vi "Test JSON Parsing.vi"() -> ()   [LabVIEW 2018, in "InfluxDB Client.lvlib"]
uses:
  InfluxDB Client.lvlib
  <vilib>/LVH/i3 JSON/i3-json.lvlib
  Classes/Client/Client.lvclass
  Classes/Results/Results.lvclass
  Classes/Result/Result.lvclass
  Classes/Series/Series.lvclass
  Controls/TagSet.ctl
panel:
  out "Values":variant[][](array[variant])
  out "Error":string
  in  "Series index":i32
  in  "Results index":i32
  out "Statement_id":i32
  out "Series name":string
  out "Result partial":bool
  out "Series partial":bool
  out "Columns":string[](array[string])
  out "Tags":T1[](array[typedef])
  out "JSON":string="{\n  \"results\": [\n    {\n      \"statement_id\": 0,\n      \"series\": [\n        {\n          \"name\": \"ChunkTest\",\n          \"columns\": [\n            \"time\",\n            \"Val\"\n          ],\n          \"values\": [\n            [\n              1.5160504613572e+18,\n              0\n            ],\n            [\n              1.5160504613732e+18,\n              1\n            ],\n            [\n              1.5160504613892e+18,\n              2\n            ],\n            [\n              1.5160504614032e+18,\n              3\n            ],\n            [\n              1.5160504614187e+18,\n              4\n            ],\n            [\n              1.5160504614347e+18,\n              5\n            ],\n            [\n              1.5160504614511e+18,\n              6\n            ],\n            [\n              1.5160504614673e+18,\n              7\n            ],\n            [\n              1.5160504614824e+18,\n              8\n            ],\n            [\n              1.5160504614985e+18,\n              9\n            ]\n          ],\n          \"partial\": true\n        }\n      ],\n      \"partial\": true\n    }\n  ]\n}"
  # "rows"
  # "columns"
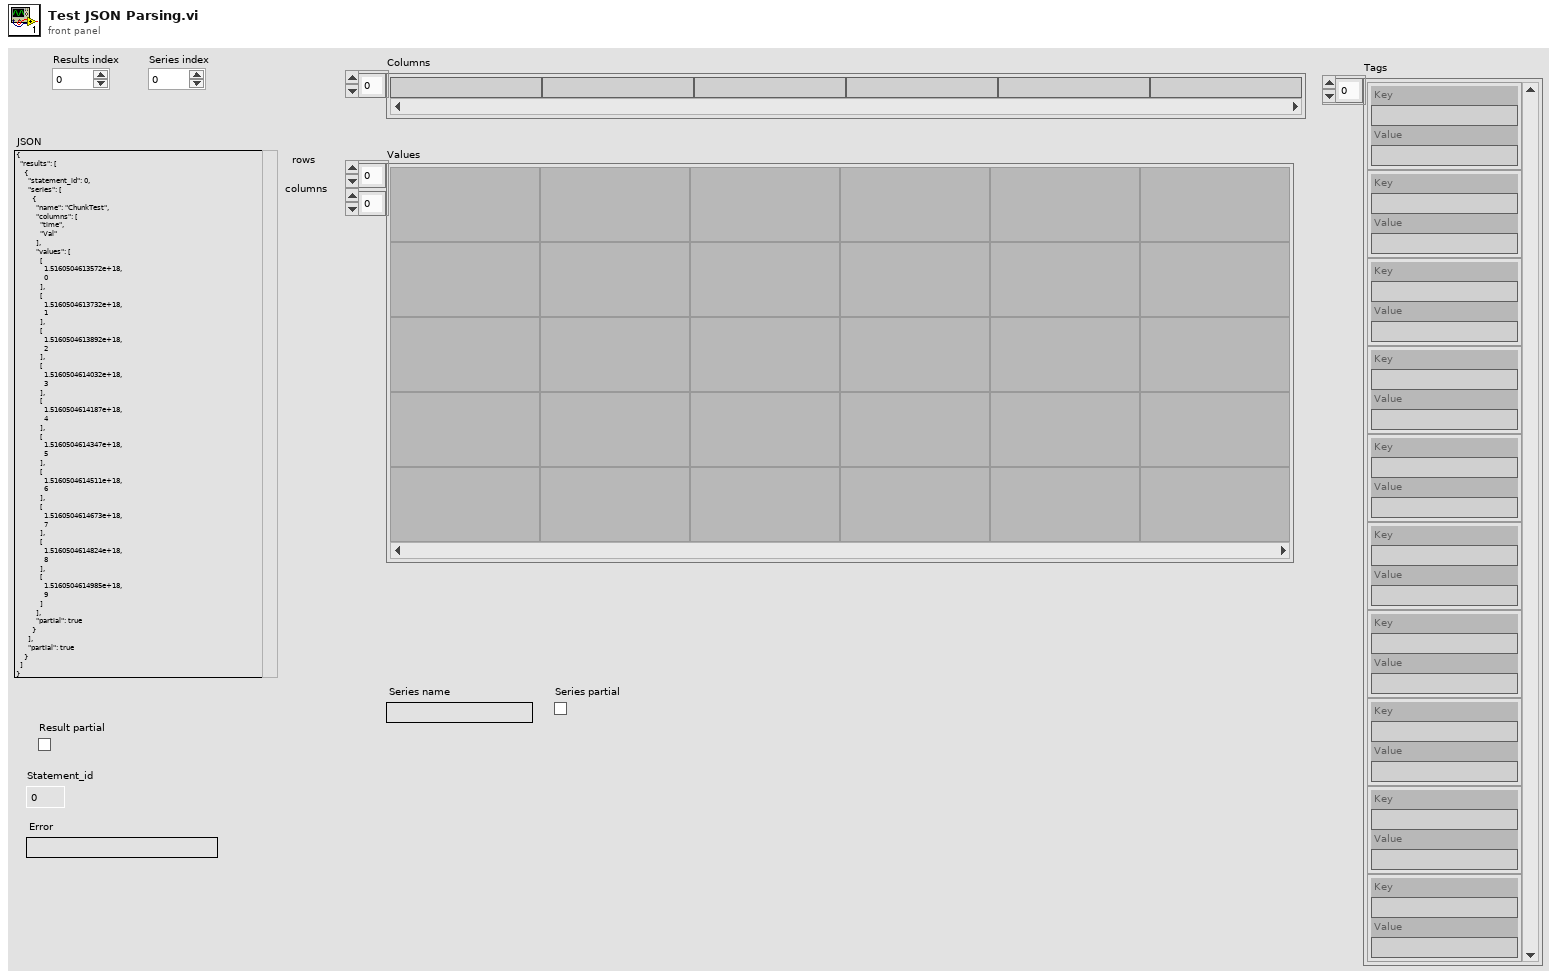
[diagram p1: front panel]
types:
  T1 = typedef "InfluxDB Client.lvlib/TagSet.ctl" = cluster{"Key":string, "Value":string}
  T2 = enum16{"open", "replace", "create", "open or create", "replace or create", "replace or create with confirmation"}
  T3 = typedef "Dictionary Object RefNum__ogtk.ctl" = refnum<k1>
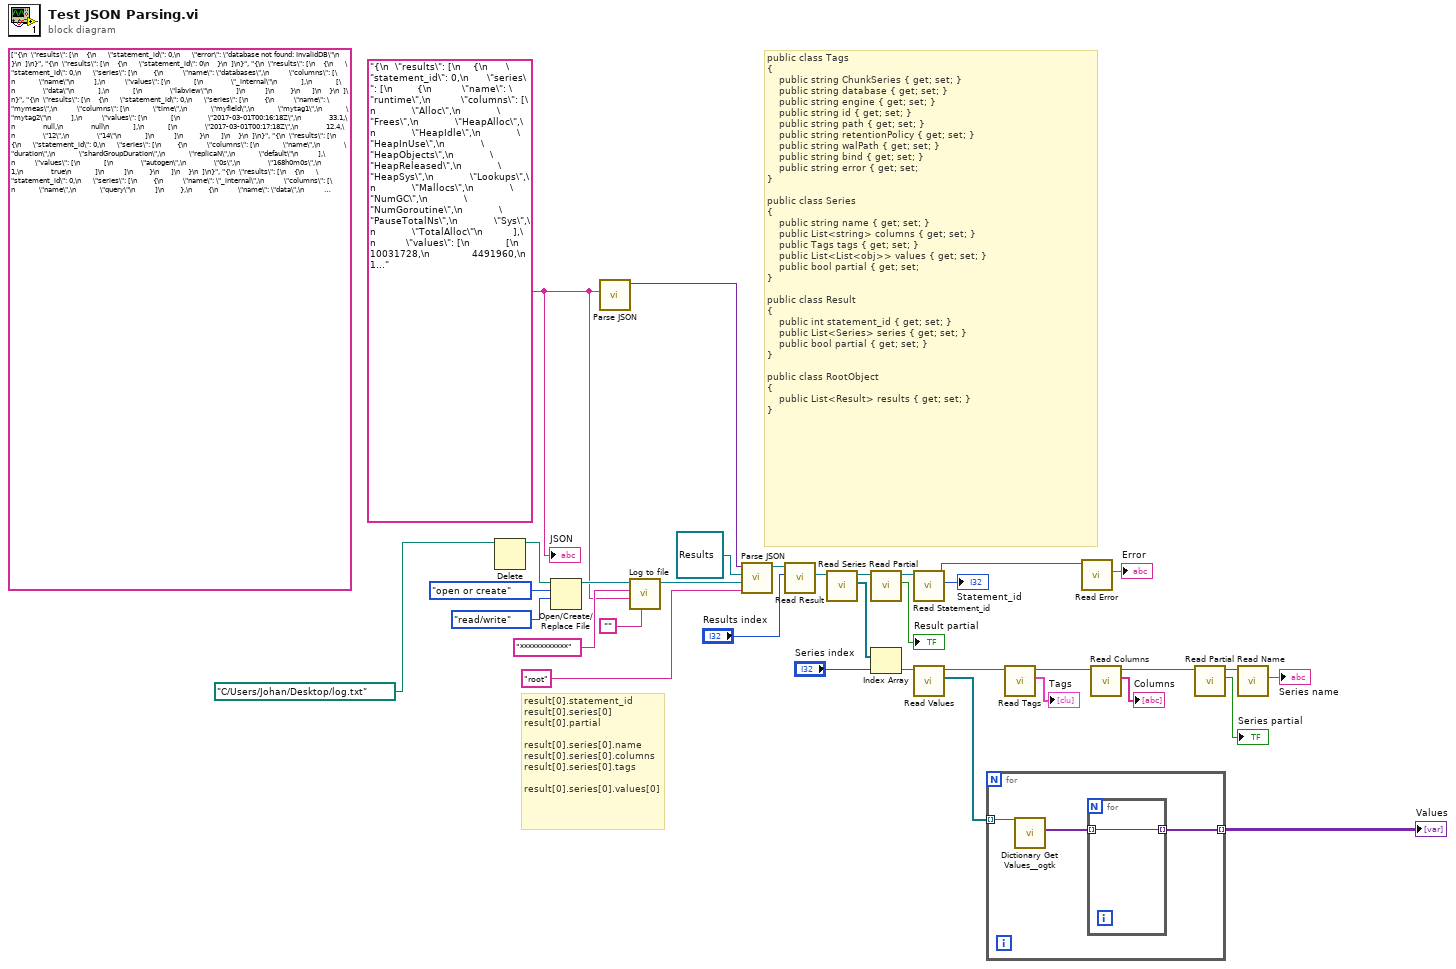
[diagram p0: block diagram]
diagram:
  w5 = "{\n  \"results\": [\n    {\n      \"statement_id\": 0,\n      \"series\": [\n        {\n          \"name\": \"runtime\",\n          \"columns\": [\n            \"Alloc\",\n            \"Frees\",\n            \"HeapAlloc\",\n            \"HeapIdle\",\n            \"HeapInUse\",\n            \"HeapObjects\",\n            \"HeapReleased\",\n            \"HeapSys\",\n            \"Lookups\",\n            \"Mallocs\",\n            \"NumGC\",\n            \"NumGoroutine\",\n            \"PauseTotalNs\",\n            \"Sys\",\n            \"TotalAlloc\"\n          ],\n          \"values\": [\n            [\n              10031728,\n              4491960,\n              10031728,\n              68689920,\n              12771328,\n              133250,\n              59473920,\n              81461248,\n              269,\n              4625210,\n              73,\n              27,\n              4009300,\n              89569528,\n              888359040\n            ]\n          ]\n        },\n        {\n          \"name\": \"queryExecutor\",\n          \"columns\": [\n            \"queriesActive\",\n            \"queriesExecuted\",\n            \"queriesFinished\",\n            \"queryDurationNs\",\n            \"recoveredPanics\"\n          ],\n          \"values\": [\n            [\n              1,\n              10,\n              9,\n              64001100,\n              0\n            ]\n          ]\n        },\n        {\n          \"name\": \"database\",\n          \"tags\": {\n            \"database\": \"_internal\"\n          },\n          \"columns\": [\n            \"numMeasurements\",\n            \"numSeries\"\n          ],\n          \"values\": [\n            [\n              12,\n              108\n            ]\n          ]\n        },\n        {\n          \"name\": \"database\",\n          \"tags\": {\n            \"database\": \"labview\"\n          },\n          \"columns\": [\n            \"numMeasurements\",\n            \"numSeries\"\n          ],\n          \"values\": [\n            [\n              1,\n              1\n            ]\n          ]\n        },\n        {\n          \"name\": \"database\",\n          \"tags\": {\n            \"database\": \"data\"\n          },\n          \"columns\": [\n            \"numMeasurements\",\n            \"numSeries\"\n          ],\n          \"values\": [\n            [\n              7,\n              23\n            ]\n          ]\n        },\n        {\n          \"name\": \"shard\",\n          \"tags\": {\n            \"database\": \"_internal\",\n            \"engine\": \"tsm1\",\n            \"id\": \"6\",\n            \"path\": \"C:\\\\Users\\\\Johan\\\\.influxdb\\\\data\\\\_internal\\\\monitor\\\\6\",\n            \"retentionPolicy\": \"monitor\",\n            \"walPath\": \"C:\\\\Users\\\\Johan\\\\.influxdb\\\\wal\\\\_internal\\\\monitor\\\\6\"\n          },\n          \"columns\": [\n            \"diskBytes\",\n            \"fieldsCreate\",\n            \"seriesCreate\",\n            \"writeBytes\",\n            \"writePointsDropped\",\n            \"writePointsErr\",\n            \"writePointsOk\",\n            \"writeReq\",\n            \"writeReqErr\",\n            \"writeReqOk\"\n          ],\n          \"values\": [\n            [\n              260046,\n              0,\n              109,\n              0,\n              0,\n              0,\n              0,\n              0,\n              0,\n              0\n            ]\n          ]\n        },\n        {\n          \"name\": \"tsm1_engine\",\n          \"tags\": {\n            \"database\": \"_internal\",\n            \"engine\": \"tsm1\",\n            \"id\": \"6\",\n            \"path\": \"C:\\\\Users\\\\Johan\\\\.influxdb\\\\data\\\\_internal\\\\monitor\\\\6\",\n            \"retentionPolicy\": \"monitor\",\n            \"walPath\": \"C:\\\\Users\\\\Johan\\\\.influxdb\\\\wal\\\\_internal\\\\monitor\\\\6\"\n          },\n          \"columns\": [\n            \"cacheCompactionDuration\",\n            \"cacheCompactionErr\",\n            \"cacheCompactions\",\n            \"cacheCompactionsActive\",\n            \"tsmFullCompactionDuration\",\n            \"tsmFullCompactionErr\",\n            \"tsmFullCompactionQueue\",\n            \"tsmFullCompactions\",\n            \"tsmFullCompactionsActive\",\n            \"tsmLevel1CompactionDuration\",\n            \"tsmLevel1CompactionErr\",\n            \"tsmLevel1CompactionQueue\",\n            \"tsmLevel1Compactions\",\n            \"tsmLevel1CompactionsActive\",\n            \"tsmLevel2CompactionDuration\",\n            \"tsmLevel2CompactionErr\",\n            \"tsmLevel2CompactionQueue\",\n            \"tsmLevel2Compactions\",\n            \"tsmLevel2CompactionsActive\",\n            \"tsmLevel3CompactionDuration\",\n            \"tsmLevel3CompactionErr\",\n            \"tsmLevel3CompactionQueue\",\n            \"tsmLevel3Compactions\",\n            \"tsmLevel3CompactionsActive\",\n            \"tsmOptimizeCompactionDuration\",\n            \"tsmOptimizeCompactionErr\",\n            \"tsmOptimizeCompactionQueue\",\n            \"tsmOptimizeCompactions\",\n            \"tsmOptimizeCompactionsActive\"\n          ],\n          \"values\": [\n            [\n              0,\n              0,\n              0,\n              0,\n              0,\n              0,\n              0,\n              0,\n              0,\n              0,\n              0,\n              0,\n              0,\n              0,\n              0,\n              0,\n              0,\n              0,\n              0,\n              0,\n              0,\n              0,\n              0,\n              0,\n              0,\n              0,\n              0,\n              0,\n              0\n            ]\n          ]\n        },\n        {\n          \"name\": \"tsm1_cache\",\n          \"tags\": {\n            \"database\": \"_internal\",\n            \"engine\": \"tsm1\",\n            \"id\": \"6\",\n            \"path\": \"C:\\\\Users\\\\Johan\\\\.influxdb\\\\data\\\\_internal\\\\monitor\\\\6\",\n            \"retentionPolicy\": \"monitor\",\n            \"walPath\": \"C:\\\\Users\\\\Johan\\\\.influxdb\\\\wal\\\\_internal\\\\monitor\\\\6\"\n          },\n          \"columns\": [\n            \"WALCompactionTimeMs\",\n            \"cacheAgeMs\",\n            \"cachedBytes\",\n            \"diskBytes\",\n            \"memBytes\",\n            \"snapshotCount\",\n            \"writeDropped\",\n            \"writeErr\",\n            \"writeOk\"\n          ],\n          \"values\": [\n            [\n              0,\n              0,\n              0,\n              0,\n              0,\n              0,\n              0,\n              0,\n              0\n            ]\n          ]\n        },\n        {\n          \"name\": \"tsm1_filestore\",\n          \"tags\": {\n            \"database\": \"_internal\",\n            \"engine\": \"tsm1\",\n            \"id\": \"6\",\n            \"path\": \"C:\\\\Users\\\\Johan\\\\.influxdb\\\\data\\\\_internal\\\\monitor\\\\6\",\n            \"retentionPolicy\": \"monitor\",\n            \"walPath\": \"C:\\\\Users\\\\Johan\\\\.influxdb\\\\wal\\\\_internal\\\\monitor\\\\6\"\n          },\n          \"columns\": [\n            \"diskBytes\",\n            \"numFiles\"\n          ],\n          \"values\": [\n            [\n              260046,\n              1\n            ]\n          ]\n        },\n        {\n          \"name\": \"tsm1_wal\",\n          \"tags\": {\n            \"database\": \"_internal\",\n            \"engine\": \"tsm1\",\n            \"id\": \"6\",\n            \"path\": \"C:\\\\Users\\\\Johan\\\\.influxdb\\\\data\\\\_internal\\\\monitor\\\\6\",\n            \"retentionPolicy\": \"monitor\",\n            \"walPath\": \"C:\\\\Users\\\\Johan\\\\.influxdb\\\\wal\\\\_internal\\\\monitor\\\\6\"\n          },\n          \"columns\": [\n            \"currentSegmentDiskBytes\",\n            \"oldSegmentsDiskBytes\",\n            \"writeErr\",\n            \"writeOk\"\n          ],\n          \"values\": [\n            [\n              0,\n              0,\n              0,\n              0\n            ]\n          ]\n        },\n        {\n          \"name\": \"shard\",\n          \"tags\": {\n            \"database\": \"data\",\n            \"engine\": \"tsm1\",\n            \"id\": \"10\",\n            \"path\": \"C:\\\\Users\\\\Johan\\\\.influxdb\\\\data\\\\data\\\\autogen\\\\10\",\n            \"retentionPolicy\": \"autogen\",\n            \"walPath\": \"C:\\\\Users\\\\Johan\\\\.influxdb\\\\wal\\\\data\\\\autogen\\\\10\"\n          },\n          \"columns\": [\n            \"diskBytes\",\n            \"fieldsCreate\",\n            \"seriesCreate\",\n            \"writeBytes\",\n            \"writePointsDropped\",\n            \"writePointsErr\",\n            \"writePointsOk\",\n            \"writeReq\",\n            \"writeReqErr\",\n            \"writeReqOk\"\n          ],\n          \"values\": [\n            [\n              614,\n              0,\n              23,\n              0,\n              0,\n              0,\n              0,\n              0,\n              0,\n              0\n            ]\n          ]\n        },\n        {\n          \"name\": \"tsm1_engine\",\n          \"tags\": {\n            \"database\": \"data\",\n            \"engine\": \"tsm1\",\n            \"id\": \"10\",\n            \"path\": \"C:\\\\Users\\\\Johan\\\\.influxdb\\\\data\\\\data\\\\autogen\\\\10\",\n            \"retentionPolicy\": \"autogen\",\n            \"walPath\": \"C:\\\\Users\\\\Johan\\\\.influxdb\\\\wal\\\\data\\\\autogen\\\\10\"\n          },\n          \"columns\": [\n            \"cacheCompactionDuration\",\n            \"cacheCompactionErr\",\n            \"cacheCompactions\",\n            \"cacheCompactionsActive\",\n            \"tsmFullCompactionDuration\",\n            \"tsmFullCompactionErr\",\n            \"tsmFullCompactionQueue\",\n            \"tsmFullCompactions\",\n            \"tsmFullCompactionsActive\",\n            \"tsmLevel1CompactionDuration\",\n            \"tsmLevel1CompactionErr\",\n            \"tsmLevel1CompactionQueue\",\n            \"tsmLevel1Compactions\",\n            \"tsmLevel1CompactionsActive\",\n            \"tsmLevel2CompactionDuration\",\n            \"tsmLevel2CompactionErr\",\n            \"tsmLevel2CompactionQueue\",\n            \"tsmLevel2Compactions\",\n            \"tsmLevel2CompactionsActive\",\n            \"tsmLevel3CompactionDuration\",\n            \"tsmLevel3CompactionErr\",\n            \"tsmLevel3CompactionQueue\",\n            \"tsmLevel3Compactions\",\n            \"tsmLevel3CompactionsActive\",\n            \"tsmOptimizeCompactionDuration\",\n            \"tsmOptimizeCompactionErr\",\n            \"tsmOptimizeCompactionQueue\",\n            \"tsmOptimizeCompactions\",\n            \"tsmOptimizeCompactionsActive\"\n          ],\n          \"values\": [\n            [\n              0,\n              0,\n              0,\n              0,\n              0,\n              0,\n              0,\n              0,\n              0,\n              0,\n              0,\n              0,\n              0,\n              0,\n              0,\n              0,\n              0,\n              0,\n              0,\n              0,\n              0,\n              0,\n              0,\n              0,\n              0,\n              0,\n              0,\n              0,\n              0\n            ]\n          ]\n        },\n        {\n          \"name\": \"tsm1_cache\",\n          \"tags\": {\n            \"database\": \"data\",\n            \"engine\": \"tsm1\",\n            \"id\": \"10\",\n            \"path\": \"C:\\\\Users\\\\Johan\\\\.influxdb\\\\data\\\\data\\\\autogen\\\\10\",\n            \"retentionPolicy\": \"autogen\",\n            \"walPath\": \"C:\\\\Users\\\\Johan\\\\.influxdb\\\\wal\\\\data\\\\autogen\\\\10\"\n          },\n          \"columns\": [\n            \"WALCompactionTimeMs\",\n            \"cacheAgeMs\",\n            \"cachedBytes\",\n            \"diskBytes\",\n            \"memBytes\",\n            \"snapshotCount\",\n            \"writeDropped\",\n            \"writeErr\",\n            \"writeOk\"\n          ],\n          \"values\": [\n            [\n              0,\n              0,\n              0,\n              0,\n              0,\n              0,\n              0,\n              0,\n              0\n            ]\n          ]\n        },\n        {\n          \"name\": \"tsm1_filestore\",\n          \"tags\": {\n            \"database\": \"data\",\n            \"engine\": \"tsm1\",\n            \"id\": \"10\",\n            \"path\": \"C:\\\\Users\\\\Johan\\\\.influxdb\\\\data\\\\data\\\\autogen\\\\10\",\n            \"retentionPolicy\": \"autogen\",\n            \"walPath\": \"C:\\\\Users\\\\Johan\\\\.influxdb\\\\wal\\\\data\\\\autogen\\\\10\"\n          },\n          \"columns\": [\n            \"diskBytes\",\n            \"numFiles\"\n          ],\n          \"values\": [\n            [\n              614,\n              1\n            ]\n          ]\n        },\n        {\n          \"name\": \"tsm1_wal\",\n          \"tags\": {\n            \"database\": \"data\",\n            \"engine\": \"tsm1\",\n            \"id\": \"10\",\n            \"path\": \"C:\\\\Users\\\\Johan\\\\.influxdb\\\\data\\\\data\\\\autogen\\\\10\",\n            \"retentionPolicy\": \"autogen\",\n            \"walPath\": \"C:\\\\Users\\\\Johan\\\\.influxdb\\\\wal\\\\data\\\\autogen\\\\10\"\n          },\n          \"columns\": [\n            \"currentSegmentDiskBytes\",\n            \"oldSegmentsDiskBytes\",\n            \"writeErr\",\n            \"writeOk\"\n          ],\n          \"values\": [\n            [\n              0,\n              0,\n              0,\n              0\n            ]\n          ]\n        },\n        {\n          \"name\": \"shard\",\n          \"tags\": {\n            \"database\": \"data\",\n            \"engine\": \"tsm1\",\n            \"id\": \"11\",\n            \"path\": \"C:\\\\Users\\\\Johan\\\\.influxdb\\\\data\\\\data\\\\autogen\\\\11\",\n            \"retentionPolicy\": \"autogen\",\n            \"walPath\": \"C:\\\\Users\\\\Johan\\\\.influxdb\\\\wal\\\\data\\\\autogen\\\\11\"\n          },\n          \"columns\": [\n            \"diskBytes\",\n            \"fieldsCreate\",\n            \"seriesCreate\",\n            \"writeBytes\",\n            \"writePointsDropped\",\n            \"writePointsErr\",\n            \"writePointsOk\",\n            \"writeReq\",\n            \"writeReqErr\",\n            \"writeReqOk\"\n          ],\n          \"values\": [\n            [\n              115,\n              0,\n              23,\n              0,\n              0,\n              0,\n              0,\n              0,\n              0,\n              0\n            ]\n          ]\n        },\n        {\n          \"name\": \"tsm1_engine\",\n          \"tags\": {\n            \"database\": \"data\",\n            \"engine\": \"tsm1\",\n            \"id\": \"11\",\n            \"path\": \"C:\\\\Users\\\\Johan\\\\.influxdb\\\\data\\\\data\\\\autogen\\\\11\",\n            \"retentionPolicy\": \"autogen\",\n            \"walPath\": \"C:\\\\Users\\\\Johan\\\\.influxdb\\\\wal\\\\data\\\\autogen\\\\11\"\n          },\n          \"columns\": [\n            \"cacheCompactionDuration\",\n            \"cacheCompactionErr\",\n            \"cacheCompactions\",\n            \"cacheCompactionsActive\",\n            \"tsmFullCompactionDuration\",\n            \"tsmFullCompactionErr\",\n            \"tsmFullCompactionQueue\",\n            \"tsmFullCompactions\",\n            \"tsmFullCompactionsActive\",\n            \"tsmLevel1CompactionDuration\",\n            \"tsmLevel1CompactionErr\",\n            \"tsmLevel1CompactionQueue\",\n            \"tsmLevel1Compactions\",\n            \"tsmLevel1CompactionsActive\",\n            \"tsmLevel2CompactionDuration\",\n            \"tsmLevel2CompactionErr\",\n            \"tsmLevel2CompactionQueue\",\n            \"tsmLevel2Compactions\",\n            \"tsmLevel2CompactionsActive\",\n            \"tsmLevel3CompactionDuration\",\n            \"tsmLevel3CompactionErr\",\n            \"tsmLevel3CompactionQueue\",\n            \"tsmLevel3Compactions\",\n            \"tsmLevel3CompactionsActive\",\n            \"tsmOptimizeCompactionDuration\",\n            \"tsmOptimizeCompactionErr\",\n            \"tsmOptimizeCompactionQueue\",\n            \"tsmOptimizeCompactions\",\n            \"tsmOptimizeCompactionsActive\"\n          ],\n          \"values\": [\n            [\n              0,\n              0,\n              0,\n              0,\n              0,\n              0,\n              0,\n              0,\n              0,\n              0,\n              0,\n              0,\n              0,\n              0,\n              0,\n              0,\n              0,\n              0,\n              0,\n              0,\n              0,\n              0,\n              0,\n              0,\n              0,\n              0,\n              0,\n              0,\n              0\n            ]\n          ]\n        },\n        {\n          \"name\": \"tsm1_cache\",\n          \"tags\": {\n            \"database\": \"data\",\n            \"engine\": \"tsm1\",\n            \"id\": \"11\",\n            \"path\": \"C:\\\\Users\\\\Johan\\\\.influxdb\\\\data\\\\data\\\\autogen\\\\11\",\n            \"retentionPolicy\": \"autogen\",\n            \"walPath\": \"C:\\\\Users\\\\Johan\\\\.influxdb\\\\wal\\\\data\\\\autogen\\\\11\"\n          },\n          \"columns\": [\n            \"WALCompactionTimeMs\",\n            \"cacheAgeMs\",\n            \"cachedBytes\",\n            \"diskBytes\",\n            \"memBytes\",\n            \"snapshotCount\",\n            \"writeDropped\",\n            \"writeErr\",\n            \"writeOk\"\n          ],\n          \"values\": [\n            [\n              0,\n              0,\n              0,\n              0,\n              0,\n              0,\n              0,\n              0,\n              0\n            ]\n          ]\n        },\n        {\n          \"name\": \"tsm1_filestore\",\n          \"tags\": {\n            \"database\": \"data\",\n            \"engine\": \"tsm1\",\n            \"id\": \"11\",\n            \"path\": \"C:\\\\Users\\\\Johan\\\\.influxdb\\\\data\\\\data\\\\autogen\\\\11\",\n            \"retentionPolicy\": \"autogen\",\n            \"walPath\": \"C:\\\\Users\\\\Johan\\\\.influxdb\\\\wal\\\\data\\\\autogen\\\\11\"\n          },\n          \"columns\": [\n            \"diskBytes\",\n            \"numFiles\"\n          ],\n          \"values\": [\n            [\n              115,\n              1\n            ]\n          ]\n        },\n        {\n          \"name\": \"tsm1_wal\",\n          \"tags\": {\n            \"database\": \"data\",\n            \"engine\": \"tsm1\",\n            \"id\": \"11\",\n            \"path\": \"C:\\\\Users\\\\Johan\\\\.influxdb\\\\data\\\\data\\\\autogen\\\\11\",\n            \"retentionPolicy\": \"autogen\",\n            \"walPath\": \"C:\\\\Users\\\\Johan\\\\.influxdb\\\\wal\\\\data\\\\autogen\\\\11\"\n          },\n          \"columns\": [\n            \"currentSegmentDiskBytes\",\n            \"oldSegmentsDiskBytes\",\n            \"writeErr\",\n            \"writeOk\"\n          ],\n          \"values\": [\n            [\n              0,\n              0,\n              0,\n              0\n            ]\n          ]\n        },\n        {\n          \"name\": \"shard\",\n          \"tags\": {\n            \"database\": \"data\",\n            \"engine\": \"tsm1\",\n            \"id\": \"12\",\n            \"path\": \"C:\\\\Users\\\\Johan\\\\.influxdb\\\\data\\\\data\\\\autogen\\\\12\",\n            \"retentionPolicy\": \"autogen\",\n            \"walPath\": \"C:\\\\Users\\\\Johan\\\\.influxdb\\\\wal\\\\data\\\\autogen\\\\12\"\n          },\n          \"columns\": [\n            \"diskBytes\",\n            \"fieldsCreate\",\n            \"seriesCreate\",\n            \"writeBytes\",\n            \"writePointsDropped\",\n            \"writePointsErr\",\n            \"writePointsOk\",\n            \"writeReq\",\n            \"writeReqErr\",\n            \"writeReqOk\"\n          ],\n          \"values\": [\n            [\n              58924,\n              0,\n              23,\n              0,\n              0,\n              0,\n              0,\n              0,\n              0,\n              0\n            ]\n          ]\n        },\n        {\n          \"name\": \"tsm1_engine\",\n          \"tags\": {\n            \"database\": \"data\",\n            \"engine\": \"tsm1\",\n            \"id\": \"12\",\n            \"path\": \"C:\\\\Users\\\\Johan\\\\.influxdb\\\\data\\\\data\\\\autogen\\\\12\",\n            \"retentionPolicy\": \"autogen\",\n            \"walPath\": \"C:\\\\Users\\\\Johan\\\\.influxdb\\\\wal\\\\data\\\\autogen\\\\12\"\n          },\n          \"columns\": [\n            \"cacheCompactionDuration\",\n            \"cacheCompactionErr\",\n            \"cacheCompactions\",\n            \"cacheCompactionsActive\",\n            \"tsmFullCompactionDuration\",\n            \"tsmFullCompactionErr\",\n            \"tsmFullCompactionQueue\",\n            \"tsmFullCompactions\",\n            \"tsmFullCompactionsActive\",\n            \"tsmLevel1CompactionDuration\",\n            \"tsmLevel1CompactionErr\",\n            \"tsmLevel1CompactionQueue\",\n            \"tsmLevel1Compactions\",\n            \"tsmLevel1CompactionsActive\",\n            \"tsmLevel2CompactionDuration\",\n            \"tsmLevel2CompactionErr\",\n            \"tsmLevel2CompactionQueue\",\n            \"tsmLevel2Compactions\",\n            \"tsmLevel2CompactionsActive\",\n            \"tsmLevel3CompactionDuration\",\n            \"tsmLevel3CompactionErr\",\n            \"tsmLevel3CompactionQueue\",\n            \"tsmLevel3Compactions\",\n            \"tsmLevel3CompactionsActive\",\n            \"tsmOptimizeCompactionDuration\",\n            \"tsmOptimizeCompactionErr\",\n            \"tsmOptimizeCompactionQueue\",\n            \"tsmOptimizeCompactions\",\n            \"tsmOptimizeCompactionsActive\"\n          ],\n          \"values\": [\n            [\n              0,\n              0,\n              0,\n              0,\n              0,\n              0,\n              0,\n              0,\n              0,\n              0,\n              0,\n              0,\n              0,\n              0,\n              0,\n              0,\n              0,\n              0,\n              0,\n              0,\n              0,\n              0,\n              0,\n              0,\n              0,\n              0,\n              0,\n              0,\n              0\n            ]\n          ]\n        },\n        {\n          \"name\": \"tsm1_cache\",\n          \"tags\": {\n            \"database\": \"data\",\n            \"engine\": \"tsm1\",\n            \"id\": \"12\",\n            \"path\": \"C:\\\\Users\\\\Johan\\\\.influxdb\\\\data\\\\data\\\\autogen\\\\12\",\n            \"retentionPolicy\": \"autogen\",\n            \"walPath\": \"C:\\\\Users\\\\Johan\\\\.influxdb\\\\wal\\\\data\\\\autogen\\\\12\"\n          },\n          \"columns\": [\n            \"WALCompactionTimeMs\",\n            \"cacheAgeMs\",\n            \"cachedBytes\",\n            \"diskBytes\",\n            \"memBytes\",\n            \"snapshotCount\",\n            \"writeDropped\",\n            \"writeErr\",\n            \"writeOk\"\n          ],\n          \"values\": [\n            [\n              0,\n              0,\n              0,\n              0,\n              0,\n              0,\n              0,\n              0,\n              0\n            ]\n          ]\n        },\n        {\n          \"name\": \"tsm1_filestore\",\n          \"tags\": {\n            \"database\": \"data\",\n            \"engine\": \"tsm1\",\n            \"id\": \"12\",\n            \"path\": \"C:\\\\Users\\\\Johan\\\\.influxdb\\\\data\\\\data\\\\autogen\\\\12\",\n            \"retentionPolicy\": \"autogen\",\n            \"walPath\": \"C:\\\\Users\\\\Johan\\\\.influxdb\\\\wal\\\\data\\\\autogen\\\\12\"\n          },\n          \"columns\": [\n            \"diskBytes\",\n            \"numFiles\"\n          ],\n          \"values\": [\n            [\n              58924,\n              1\n            ]\n          ]\n        },\n        {\n          \"name\": \"tsm1_wal\",\n          \"tags\": {\n            \"database\": \"data\",\n            \"engine\": \"tsm1\",\n            \"id\": \"12\",\n            \"path\": \"C:\\\\Users\\\\Johan\\\\.influxdb\\\\data\\\\data\\\\autogen\\\\12\",\n            \"retentionPolicy\": \"autogen\",\n            \"walPath\": \"C:\\\\Users\\\\Johan\\\\.influxdb\\\\wal\\\\data\\\\autogen\\\\12\"\n          },\n          \"columns\": [\n            \"currentSegmentDiskBytes\",\n            \"oldSegmentsDiskBytes\",\n            \"writeErr\",\n            \"writeOk\"\n          ],\n          \"values\": [\n            [\n              0,\n              0,\n              0,\n              0\n            ]\n          ]\n        },\n        {\n          \"name\": \"shard\",\n          \"tags\": {\n            \"database\": \"_internal\",\n            \"engine\": \"tsm1\",\n            \"id\": \"13\",\n            \"path\": \"C:\\\\Users\\\\Johan\\\\.influxdb\\\\data\\\\_internal\\\\monitor\\\\13\",\n            \"retentionPolicy\": \"monitor\",\n            \"walPath\": \"C:\\\\Users\\\\Johan\\\\.influxdb\\\\wal\\\\_internal\\\\monitor\\\\13\"\n          },\n          \"columns\": [\n            \"diskBytes\",\n            \"fieldsCreate\",\n            \"seriesCreate\",\n            \"writeBytes\",\n            \"writePointsDropped\",\n            \"writePointsErr\",\n            \"writePointsOk\",\n            \"writeReq\",\n            \"writeReqErr\",\n            \"writeReqOk\"\n          ],\n          \"values\": [\n            [\n              157086,\n              0,\n              109,\n              0,\n              0,\n              0,\n              0,\n              0,\n              0,\n              0\n            ]\n          ]\n        },\n        {\n          \"name\": \"tsm1_engine\",\n          \"tags\": {\n            \"database\": \"_internal\",\n            \"engine\": \"tsm1\",\n            \"id\": \"13\",\n            \"path\": \"C:\\\\Users\\\\Johan\\\\.influxdb\\\\data\\\\_internal\\\\monitor\\\\13\",\n            \"retentionPolicy\": \"monitor\",\n            \"walPath\": \"C:\\\\Users\\\\Johan\\\\.influxdb\\\\wal\\\\_internal\\\\monitor\\\\13\"\n          },\n          \"columns\": [\n            \"cacheCompactionDuration\",\n            \"cacheCompactionErr\",\n            \"cacheCompactions\",\n            \"cacheCompactionsActive\",\n            \"tsmFullCompactionDuration\",\n            \"tsmFullCompactionErr\",\n            \"tsmFullCompactionQueue\",\n            \"tsmFullCompactions\",\n            \"tsmFullCompactionsActive\",\n            \"tsmLevel1CompactionDuration\",\n            \"tsmLevel1CompactionErr\",\n            \"tsmLevel1CompactionQueue\",\n            \"tsmLevel1Compactions\",\n            \"tsmLevel1CompactionsActive\",\n            \"tsmLevel2CompactionDuration\",\n            \"tsmLevel2CompactionErr\",\n            \"tsmLevel2CompactionQueue\",\n            \"tsmLevel2Compactions\",\n            \"tsmLevel2CompactionsActive\",\n            \"tsmLevel3CompactionDuration\",\n            \"tsmLevel3CompactionErr\",\n            \"tsmLevel3CompactionQueue\",\n            \"tsmLevel3Compactions\",\n            \"tsmLevel3CompactionsActive\",\n            \"tsmOptimizeCompactionDuration\",\n            \"tsmOptimizeCompactionErr\",\n            \"tsmOptimizeCompactionQueue\",\n            \"tsmOptimizeCompactions\",\n            \"tsmOptimizeCompactionsActive\"\n          ],\n          \"values\": [\n            [\n              0,\n              0,\n              0,\n              0,\n              0,\n              0,\n              0,\n              0,\n              0,\n              0,\n              0,\n              0,\n              0,\n              0,\n              0,\n              0,\n              0,\n              0,\n              0,\n              0,\n              0,\n              0,\n              0,\n              0,\n              0,\n              0,\n              0,\n              0,\n              0\n            ]\n          ]\n        },\n        {\n          \"name\": \"tsm1_cache\",\n          \"tags\": {\n            \"database\": \"_internal\",\n            \"engine\": \"tsm1\",\n            \"id\": \"13\",\n            \"path\": \"C:\\\\Users\\\\Johan\\\\.influxdb\\\\data\\\\_internal\\\\monitor\\\\13\",\n            \"retentionPolicy\": \"monitor\",\n            \"walPath\": \"C:\\\\Users\\\\Johan\\\\.influxdb\\\\wal\\\\_internal\\\\monitor\\\\13\"\n          },\n          \"columns\": [\n            \"WALCompactionTimeMs\",\n            \"cacheAgeMs\",\n            \"cachedBytes\",\n            \"diskBytes\",\n            \"memBytes\",\n            \"snapshotCount\",\n            \"writeDropped\",\n            \"writeErr\",\n            \"writeOk\"\n          ],\n          \"values\": [\n            [\n              0,\n              0,\n              0,\n              0,\n              0,\n              0,\n              0,\n              0,\n              0\n            ]\n          ]\n        },\n        {\n          \"name\": \"tsm1_filestore\",\n          \"tags\": {\n            \"database\": \"_internal\",\n            \"engine\": \"tsm1\",\n            \"id\": \"13\",\n            \"path\": \"C:\\\\Users\\\\Johan\\\\.influxdb\\\\data\\\\_internal\\\\monitor\\\\13\",\n            \"retentionPolicy\": \"monitor\",\n            \"walPath\": \"C:\\\\Users\\\\Johan\\\\.influxdb\\\\wal\\\\_internal\\\\monitor\\\\13\"\n          },\n          \"columns\": [\n            \"diskBytes\",\n            \"numFiles\"\n          ],\n          \"values\": [\n            [\n              157086,\n              1\n            ]\n          ]\n        },\n        {\n          \"name\": \"tsm1_wal\",\n          \"tags\": {\n            \"database\": \"_internal\",\n            \"engine\": \"tsm1\",\n            \"id\": \"13\",\n            \"path\": \"C:\\\\Users\\\\Johan\\\\.influxdb\\\\data\\\\_internal\\\\monitor\\\\13\",\n            \"retentionPolicy\": \"monitor\",\n            \"walPath\": \"C:\\\\Users\\\\Johan\\\\.influxdb\\\\wal\\\\_internal\\\\monitor\\\\13\"\n          },\n          \"columns\": [\n            \"currentSegmentDiskBytes\",\n            \"oldSegmentsDiskBytes\",\n            \"writeErr\",\n            \"writeOk\"\n          ],\n          \"values\": [\n            [\n              0,\n              0,\n              0,\n              0\n            ]\n          ]\n        },\n        {\n          \"name\": \"shard\",\n          \"tags\": {\n            \"database\": \"_internal\",\n            \"engine\": \"tsm1\",\n            \"id\": \"14\",\n            \"path\": \"C:\\\\Users\\\\Johan\\\\.influxdb\\\\data\\\\_internal\\\\monitor\\\\14\",\n            \"retentionPolicy\": \"monitor\",\n            \"walPath\": \"C:\\\\Users\\\\Johan\\\\.influxdb\\\\wal\\\\_internal\\\\monitor\\\\14\"\n          },\n          \"columns\": [\n            \"diskBytes\",\n            \"fieldsCreate\",\n            \"seriesCreate\",\n            \"writeBytes\",\n            \"writePointsDropped\",\n            \"writePointsErr\",\n            \"writePointsOk\",\n            \"writeReq\",\n            \"writeReqErr\",\n            \"writeReqOk\"\n          ],\n          \"values\": [\n            [\n              306311,\n              0,\n              109,\n              0,\n              0,\n              0,\n              0,\n              0,\n              0,\n              0\n            ]\n          ]\n        },\n        {\n          \"name\": \"tsm1_engine\",\n          \"tags\": {\n            \"database\": \"_internal\",\n            \"engine\": \"tsm1\",\n            \"id\": \"14\",\n            \"path\": \"C:\\\\Users\\\\Johan\\\\.influxdb\\\\data\\\\_internal\\\\monitor\\\\14\",\n            \"retentionPolicy\": \"monitor\",\n            \"walPath\": \"C:\\\\Users\\\\Johan\\\\.influxdb\\\\wal\\\\_internal\\\\monitor\\\\14\"\n          },\n          \"columns\": [\n            \"cacheCompactionDuration\",\n            \"cacheCompactionErr\",\n            \"cacheCompactions\",\n            \"cacheCompactionsActive\",\n            \"tsmFullCompactionDuration\",\n            \"tsmFullCompactionErr\",\n            \"tsmFullCompactionQueue\",\n            \"tsmFullCompactions\",\n            \"tsmFullCompactionsActive\",\n            \"tsmLevel1CompactionDuration\",\n            \"tsmLevel1CompactionErr\",\n            \"tsmLevel1CompactionQueue\",\n            \"tsmLevel1Compactions\",\n            \"tsmLevel1CompactionsActive\",\n            \"tsmLevel2CompactionDuration\",\n            \"tsmLevel2CompactionErr\",\n            \"tsmLevel2CompactionQueue\",\n            \"tsmLevel2Compactions\",\n            \"tsmLevel2CompactionsActive\",\n            \"tsmLevel3CompactionDuration\",\n            \"tsmLevel3CompactionErr\",\n            \"tsmLevel3CompactionQueue\",\n            \"tsmLevel3Compactions\",\n            \"tsmLevel3CompactionsActive\",\n            \"tsmOptimizeCompactionDuration\",\n            \"tsmOptimizeCompactionErr\",\n            \"tsmOptimizeCompactionQueue\",\n            \"tsmOptimizeCompactions\",\n            \"tsmOptimizeCompactionsActive\"\n          ],\n          \"values\": [\n            [\n              0,\n              0,\n              0,\n              0,\n              0,\n              0,\n              0,\n              0,\n              0,\n              0,\n              0,\n              0,\n              0,\n              0,\n              0,\n              0,\n              0,\n              0,\n              0,\n              0,\n              0,\n              0,\n              0,\n              0,\n              0,\n              0,\n              0,\n              0,\n              0\n            ]\n          ]\n        },\n        {\n          \"name\": \"tsm1_cache\",\n          \"tags\": {\n            \"database\": \"_internal\",\n            \"engine\": \"tsm1\",\n            \"id\": \"14\",\n            \"path\": \"C:\\\\Users\\\\Johan\\\\.influxdb\\\\data\\\\_internal\\\\monitor\\\\14\",\n            \"retentionPolicy\": \"monitor\",\n            \"walPath\": \"C:\\\\Users\\\\Johan\\\\.influxdb\\\\wal\\\\_internal\\\\monitor\\\\14\"\n          },\n          \"columns\": [\n            \"WALCompactionTimeMs\",\n            \"cacheAgeMs\",\n            \"cachedBytes\",\n            \"diskBytes\",\n            \"memBytes\",\n            \"snapshotCount\",\n            \"writeDropped\",\n            \"writeErr\",\n            \"writeOk\"\n          ],\n          \"values\": [\n            [\n              0,\n              0,\n              0,\n              0,\n              0,\n              0,\n              0,\n              0,\n              0\n            ]\n          ]\n        },\n        {\n          \"name\": \"tsm1_filestore\",\n          \"tags\": {\n            \"database\": \"_internal\",\n            \"engine\": \"tsm1\",\n            \"id\": \"14\",\n            \"path\": \"C:\\\\Users\\\\Johan\\\\.influxdb\\\\data\\\\_internal\\\\monitor\\\\14\",\n            \"retentionPolicy\": \"monitor\",\n            \"walPath\": \"C:\\\\Users\\\\Johan\\\\.influxdb\\\\wal\\\\_internal\\\\monitor\\\\14\"\n          },\n          \"columns\": [\n            \"diskBytes\",\n            \"numFiles\"\n          ],\n          \"values\": [\n            [\n              306311,\n              1\n            ]\n          ]\n        },\n        {\n          \"name\": \"tsm1_wal\",\n          \"tags\": {\n            \"database\": \"_internal\",\n            \"engine\": \"tsm1\",\n            \"id\": \"14\",\n            \"path\": \"C:\\\\Users\\\\Johan\\\\.influxdb\\\\data\\\\_internal\\\\monitor\\\\14\",\n            \"retentionPolicy\": \"monitor\",\n            \"walPath\": \"C:\\\\Users\\\\Johan\\\\.influxdb\\\\wal\\\\_internal\\\\monitor\\\\14\"\n          },\n          \"columns\": [\n            \"currentSegmentDiskBytes\",\n            \"oldSegmentsDiskBytes\",\n            \"writeErr\",\n            \"writeOk\"\n          ],\n          \"values\": [\n            [\n              0,\n              0,\n              0,\n              0\n            ]\n          ]\n        },\n        {\n          \"name\": \"shard\",\n          \"tags\": {\n            \"database\": \"_internal\",\n            \"engine\": \"tsm1\",\n            \"id\": \"15\",\n            \"path\": \"C:\\\\Users\\\\Johan\\\\.influxdb\\\\data\\\\_internal\\\\monitor\\\\15\",\n            \"retentionPolicy\": \"monitor\",\n            \"walPath\": \"C:\\\\Users\\\\Johan\\\\.influxdb\\\\wal\\\\_internal\\\\monitor\\\\15\"\n          },\n          \"columns\": [\n            \"diskBytes\",\n            \"fieldsCreate\",\n            \"seriesCreate\",\n            \"writeBytes\",\n            \"writePointsDropped\",\n            \"writePointsErr\",\n            \"writePointsOk\",\n            \"writeReq\",\n            \"writeReqErr\",\n            \"writeReqOk\"\n          ],\n          \"values\": [\n            [\n              697298,\n              0,\n              109,\n              0,\n              0,\n              0,\n              0,\n              0,\n              0,\n              0\n            ]\n          ]\n        },\n        {\n          \"name\": \"tsm1_engine\",\n          \"tags\": {\n            \"database\": \"_internal\",\n            \"engine\": \"tsm1\",\n            \"id\": \"15\",\n            \"path\": \"C:\\\\Users\\\\Johan\\\\.influxdb\\\\data\\\\_internal\\\\monitor\\\\15\",\n            \"retentionPolicy\": \"monitor\",\n            \"walPath\": \"C:\\\\Users\\\\Johan\\\\.influxdb\\\\wal\\\\_internal\\\\monitor\\\\15\"\n          },\n          \"columns\": [\n            \"cacheCompactionDuration\",\n            \"cacheCompactionErr\",\n            \"cacheCompactions\",\n            \"cacheCompactionsActive\",\n            \"tsmFullCompactionDuration\",\n            \"tsmFullCompactionErr\",\n            \"tsmFullCompactionQueue\",\n            \"tsmFullCompactions\",\n            \"tsmFullCompactionsActive\",\n            \"tsmLevel1CompactionDuration\",\n            \"tsmLevel1CompactionErr\",\n            \"tsmLevel1CompactionQueue\",\n            \"tsmLevel1Compactions\",\n            \"tsmLevel1CompactionsActive\",\n            \"tsmLevel2CompactionDuration\",\n            \"tsmLevel2CompactionErr\",\n            \"tsmLevel2CompactionQueue\",\n            \"tsmLevel2Compactions\",\n            \"tsmLevel2CompactionsActive\",\n            \"tsmLevel3CompactionDuration\",\n            \"tsmLevel3CompactionErr\",\n            \"tsmLevel3CompactionQueue\",\n            \"tsmLevel3Compactions\",\n            \"tsmLevel3CompactionsActive\",\n            \"tsmOptimizeCompactionDuration\",\n            \"tsmOptimizeCompactionErr\",\n            \"tsmOptimizeCompactionQueue\",\n            \"tsmOptimizeCompactions\",\n            \"tsmOptimizeCompactionsActive\"\n          ],\n          \"values\": [\n            [\n              0,\n              0,\n              0,\n              0,\n              0,\n              0,\n              0,\n              0,\n              0,\n              0,\n              0,\n              0,\n              0,\n              0,\n              0,\n              0,\n              0,\n              0,\n              0,\n              0,\n              0,\n              0,\n              0,\n              0,\n              0,\n              0,\n              0,\n              0,\n              0\n            ]\n          ]\n        },\n        {\n          \"name\": \"tsm1_cache\",\n          \"tags\": {\n            \"database\": \"_internal\",\n            \"engine\": \"tsm1\",\n            \"id\": \"15\",\n            \"path\": \"C:\\\\Users\\\\Johan\\\\.influxdb\\\\data\\\\_internal\\\\monitor\\\\15\",\n            \"retentionPolicy\": \"monitor\",\n            \"walPath\": \"C:\\\\Users\\\\Johan\\\\.influxdb\\\\wal\\\\_internal\\\\monitor\\\\15\"\n          },\n          \"columns\": [\n            \"WALCompactionTimeMs\",\n            \"cacheAgeMs\",\n            \"cachedBytes\",\n            \"diskBytes\",\n            \"memBytes\",\n            \"snapshotCount\",\n            \"writeDropped\",\n            \"writeErr\",\n            \"writeOk\"\n          ],\n          \"values\": [\n            [\n              0,\n              1416518,\n              0,\n              0,\n              0,\n              0,\n              0,\n              0,\n              0\n            ]\n          ]\n        },\n        {\n          \"name\": \"tsm1_filestore\",\n          \"tags\": {\n            \"database\": \"_internal\",\n            \"engine\": \"tsm1\",\n            \"id\": \"15\",\n            \"path\": \"C:\\\\Users\\\\Johan\\\\.influxdb\\\\data\\\\_internal\\\\monitor\\\\15\",\n            \"retentionPolicy\": \"monitor\",\n            \"walPath\": \"C:\\\\Users\\\\Johan\\\\.influxdb\\\\wal\\\\_internal\\\\monitor\\\\15\"\n          },\n          \"columns\": [\n            \"diskBytes\",\n            \"numFiles\"\n          ],\n          \"values\": [\n            [\n              697298,\n              2\n            ]\n          ]\n        },\n        {\n          \"name\": \"tsm1_wal\",\n          \"tags\": {\n            \"database\": \"_internal\",\n            \"engine\": \"tsm1\",\n            \"id\": \"15\",\n            \"path\": \"C:\\\\Users\\\\Johan\\\\.influxdb\\\\data\\\\_internal\\\\monitor\\\\15\",\n            \"retentionPolicy\": \"monitor\",\n            \"walPath\": \"C:\\\\Users\\\\Johan\\\\.influxdb\\\\wal\\\\_internal\\\\monitor\\\\15\"\n          },\n          \"columns\": [\n            \"currentSegmentDiskBytes\",\n            \"oldSegmentsDiskBytes\",\n            \"writeErr\",\n            \"writeOk\"\n          ],\n          \"values\": [\n            [\n              0,\n              0,\n              0,\n              0\n            ]\n          ]\n        },\n        {\n          \"name\": \"shard\",\n          \"tags\": {\n            \"database\": \"data\",\n            \"engine\": \"tsm1\",\n            \"id\": \"16\",\n            \"path\": \"C:\\\\Users\\\\Johan\\\\.influxdb\\\\data\\\\data\\\\autogen\\\\16\",\n            \"retentionPolicy\": \"autogen\",\n            \"walPath\": \"C:\\\\Users\\\\Johan\\\\.influxdb\\\\wal\\\\data\\\\autogen\\\\16\"\n          },\n          \"columns\": [\n            \"diskBytes\",\n            \"fieldsCreate\",\n            \"seriesCreate\",\n            \"writeBytes\",\n            \"writePointsDropped\",\n            \"writePointsErr\",\n            \"writePointsOk\",\n            \"writeReq\",\n            \"writeReqErr\",\n            \"writeReqOk\"\n          ],\n          \"values\": [\n            [\n              370,\n              0,\n              23,\n              0,\n              0,\n              0,\n              0,\n              0,\n              0,\n              0\n            ]\n          ]\n        },\n        {\n          \"name\": \"tsm1_engine\",\n          \"tags\": {\n            \"database\": \"data\",\n            \"engine\": \"tsm1\",\n            \"id\": \"16\",\n            \"path\": \"C:\\\\Users\\\\Johan\\\\.influxdb\\\\data\\\\data\\\\autogen\\\\16\",\n            \"retentionPolicy\": \"autogen\",\n            \"walPath\": \"C:\\\\Users\\\\Johan\\\\.influxdb\\\\wal\\\\data\\\\autogen\\\\16\"\n          },\n          \"columns\": [\n            \"cacheCompactionDuration\",\n            \"cacheCompactionErr\",\n            \"cacheCompactions\",\n            \"cacheCompactionsActive\",\n            \"tsmFullCompactionDuration\",\n            \"tsmFullCompactionErr\",\n            \"tsmFullCompactionQueue\",\n            \"tsmFullCompactions\",\n            \"tsmFullCompactionsActive\",\n            \"tsmLevel1CompactionDuration\",\n            \"tsmLevel1CompactionErr\",\n            \"tsmLevel1CompactionQueue\",\n            \"tsmLevel1Compactions\",\n            \"tsmLevel1CompactionsActive\",\n            \"tsmLevel2CompactionDuration\",\n            \"tsmLevel2CompactionErr\",\n            \"tsmLevel2CompactionQueue\",\n            \"tsmLevel2Compactions\",\n            \"tsmLevel2CompactionsActive\",\n            \"tsmLevel3CompactionDuration\",\n            \"tsmLevel3CompactionErr\",\n            \"tsmLevel3CompactionQueue\",\n            \"tsmLevel3Compactions\",\n            \"tsmLevel3CompactionsActive\",\n            \"tsmOptimizeCompactionDuration\",\n            \"tsmOptimizeCompactionErr\",\n            \"tsmOptimizeCompactionQueue\",\n            \"tsmOptimizeCompactions\",\n            \"tsmOptimizeCompactionsActive\"\n          ],\n          \"values\": [\n            [\n              0,\n              0,\n              0,\n              0,\n              0,\n              0,\n              0,\n              0,\n              0,\n              0,\n              0,\n              0,\n              0,\n              0,\n              0,\n              0,\n              0,\n              0,\n              0,\n              0,\n              0,\n              0,\n              0,\n              0,\n              0,\n              0,\n              0,\n              0,\n              0\n            ]\n          ]\n        },\n        {\n          \"name\": \"tsm1_cache\",\n          \"tags\": {\n            \"database\": \"data\",\n            \"engine\": \"tsm1\",\n            \"id\": \"16\",\n            \"path\": \"C:\\\\Users\\\\Johan\\\\.influxdb\\\\data\\\\data\\\\autogen\\\\16\",\n            \"retentionPolicy\": \"autogen\",\n            \"walPath\": \"C:\\\\Users\\\\Johan\\\\.influxdb\\\\wal\\\\data\\\\autogen\\\\16\"\n          },\n          \"columns\": [\n            \"WALCompactionTimeMs\",\n            \"cacheAgeMs\",\n            \"cachedBytes\",\n            \"diskBytes\",\n            \"memBytes\",\n            \"snapshotCount\",\n            \"writeDropped\",\n            \"writeErr\",\n            \"writeOk\"\n          ],\n          \"values\": [\n            [\n              0,\n              0,\n              0,\n              0,\n              0,\n              0,\n              0,\n              0,\n              0\n            ]\n          ]\n        },\n        {\n          \"name\": \"tsm1_filestore\",\n          \"tags\": {\n            \"database\": \"data\",\n            \"engine\": \"tsm1\",\n            \"id\": \"16\",\n            \"path\": \"C:\\\\Users\\\\Johan\\\\.influxdb\\\\data\\\\data\\\\autogen\\\\16\",\n            \"retentionPolicy\": \"autogen\",\n            \"walPath\": \"C:\\\\Users\\\\Johan\\\\.influxdb\\\\wal\\\\data\\\\autogen\\\\16\"\n          },\n          \"columns\": [\n            \"diskBytes\",\n            \"numFiles\"\n          ],\n          \"values\": [\n            [\n              370,\n              1\n            ]\n          ]\n        },\n        {\n          \"name\": \"tsm1_wal\",\n          \"tags\": {\n            \"database\": \"data\",\n            \"engine\": \"tsm1\",\n            \"id\": \"16\",\n            \"path\": \"C:\\\\Users\\\\Johan\\\\.influxdb\\\\data\\\\data\\\\autogen\\\\16\",\n            \"retentionPolicy\": \"autogen\",\n            \"walPath\": \"C:\\\\Users\\\\Johan\\\\.influxdb\\\\wal\\\\data\\\\autogen\\\\16\"\n          },\n          \"columns\": [\n            \"currentSegmentDiskBytes\",\n            \"oldSegmentsDiskBytes\",\n            \"writeErr\",\n            \"writeOk\"\n          ],\n          \"values\": [\n            [\n              0,\n              0,\n              0,\n              0\n            ]\n          ]\n        },\n        {\n          \"name\": \"shard\",\n          \"tags\": {\n            \"database\": \"data\",\n            \"engine\": \"tsm1\",\n            \"id\": \"17\",\n            \"path\": \"C:\\\\Users\\\\Johan\\\\.influxdb\\\\data\\\\data\\\\autogen\\\\17\",\n            \"retentionPolicy\": \"autogen\",\n            \"walPath\": \"C:\\\\Users\\\\Johan\\\\.influxdb\\\\wal\\\\data\\\\autogen\\\\17\"\n          },\n          \"columns\": [\n            \"diskBytes\",\n            \"fieldsCreate\",\n            \"seriesCreate\",\n            \"writeBytes\",\n            \"writePointsDropped\",\n            \"writePointsErr\",\n            \"writePointsOk\",\n            \"writeReq\",\n            \"writeReqErr\",\n            \"writeReqOk\"\n          ],\n          \"values\": [\n            [\n              264,\n              0,\n              23,\n              0,\n              0,\n              0,\n              0,\n              0,\n              0,\n              0\n            ]\n          ]\n        },\n        {\n          \"name\": \"tsm1_engine\",\n          \"tags\": {\n            \"database\": \"data\",\n            \"engine\": \"tsm1\",\n            \"id\": \"17\",\n            \"path\": \"C:\\\\Users\\\\Johan\\\\.influxdb\\\\data\\\\data\\\\autogen\\\\17\",\n            \"retentionPolicy\": \"autogen\",\n            \"walPath\": \"C:\\\\Users\\\\Johan\\\\.influxdb\\\\wal\\\\data\\\\autogen\\\\17\"\n          },\n          \"columns\": [\n            \"cacheCompactionDuration\",\n            \"cacheCompactionErr\",\n            \"cacheCompactions\",\n            \"cacheCompactionsActive\",\n            \"tsmFullCompactionDuration\",\n            \"tsmFullCompactionErr\",\n            \"tsmFullCompactionQueue\",\n            \"tsmFullCompactions\",\n            \"tsmFullCompactionsActive\",\n            \"tsmLevel1CompactionDuration\",\n            \"tsmLevel1CompactionErr\",\n            \"tsmLevel1CompactionQueue\",\n            \"tsmLevel1Compactions\",\n            \"tsmLevel1CompactionsActive\",\n            \"tsmLevel2CompactionDuration\",\n            \"tsmLevel2CompactionErr\",\n            \"tsmLevel2CompactionQueue\",\n            \"tsmLevel2Compactions\",\n            \"tsmLevel2CompactionsActive\",\n            \"tsmLevel3CompactionDuration\",\n            \"tsmLevel3CompactionErr\",\n            \"tsmLevel3CompactionQueue\",\n            \"tsmLevel3Compactions\",\n            \"tsmLevel3CompactionsActive\",\n            \"tsmOptimizeCompactionDuration\",\n            \"tsmOptimizeCompactionErr\",\n            \"tsmOptimizeCompactionQueue\",\n            \"tsmOptimizeCompactions\",\n            \"tsmOptimizeCompactionsActive\"\n          ],\n          \"values\": [\n            [\n              0,\n              0,\n              0,\n              0,\n              0,\n              0,\n              0,\n              0,\n              0,\n              0,\n              0,\n              0,\n              0,\n              0,\n              0,\n              0,\n              0,\n              0,\n              0,\n              0,\n              0,\n              0,\n              0,\n              0,\n              0,\n              0,\n              0,\n              0,\n              0\n            ]\n          ]\n        },\n        {\n          \"name\": \"tsm1_cache\",\n          \"tags\": {\n            \"database\": \"data\",\n            \"engine\": \"tsm1\",\n            \"id\": \"17\",\n            \"path\": \"C:\\\\Users\\\\Johan\\\\.influxdb\\\\data\\\\data\\\\autogen\\\\17\",\n            \"retentionPolicy\": \"autogen\",\n            \"walPath\": \"C:\\\\Users\\\\Johan\\\\.influxdb\\\\wal\\\\data\\\\autogen\\\\17\"\n          },\n          \"columns\": [\n            \"WALCompactionTimeMs\",\n            \"cacheAgeMs\",\n            \"cachedBytes\",\n            \"diskBytes\",\n            \"memBytes\",\n            \"snapshotCount\",\n            \"writeDropped\",\n            \"writeErr\",\n            \"writeOk\"\n          ],\n          \"values\": [\n            [\n              0,\n              0,\n              0,\n              0,\n              0,\n              0,\n              0,\n              0,\n              0\n            ]\n          ]\n        },\n        {\n          \"name\": \"tsm1_filestore\",\n          \"tags\": {\n            \"database\": \"data\",\n            \"engine\": \"tsm1\",\n            \"id\": \"17\",\n            \"path\": \"C:\\\\Users\\\\Johan\\\\.influxdb\\\\data\\\\data\\\\autogen\\\\17\",\n            \"retentionPolicy\": \"autogen\",\n            \"walPath\": \"C:\\\\Users\\\\Johan\\\\.influxdb\\\\wal\\\\data\\\\autogen\\\\17\"\n          },\n          \"columns\": [\n            \"diskBytes\",\n            \"numFiles\"\n          ],\n          \"values\": [\n            [\n              264,\n              1\n            ]\n          ]\n        },\n        {\n          \"name\": \"tsm1_wal\",\n          \"tags\": {\n            \"database\": \"data\",\n            \"engine\": \"tsm1\",\n            \"id\": \"17\",\n            \"path\": \"C:\\\\Users\\\\Johan\\\\.influxdb\\\\data\\\\data\\\\autogen\\\\17\",\n            \"retentionPolicy\": \"autogen\",\n            \"walPath\": \"C:\\\\Users\\\\Johan\\\\.influxdb\\\\wal\\\\data\\\\autogen\\\\17\"\n          },\n          \"columns\": [\n            \"currentSegmentDiskBytes\",\n            \"oldSegmentsDiskBytes\",\n            \"writeErr\",\n            \"writeOk\"\n          ],\n          \"values\": [\n            [\n              0,\n              0,\n              0,\n              0\n            ]\n          ]\n        },\n        {\n          \"name\": \"shard\",\n          \"tags\": {\n            \"database\": \"labview\",\n            \"engine\": \"tsm1\",\n            \"id\": \"20\",\n            \"path\": \"C:\\\\Users\\\\Johan\\\\.influxdb\\\\data\\\\labview\\\\autogen\\\\20\",\n            \"retentionPolicy\": \"autogen\",\n            \"walPath\": \"C:\\\\Users\\\\Johan\\\\.influxdb\\\\wal\\\\labview\\\\autogen\\\\20\"\n          },\n          \"columns\": [\n            \"diskBytes\",\n            \"fieldsCreate\",\n            \"seriesCreate\",\n            \"writeBytes\",\n            \"writePointsDropped\",\n            \"writePointsErr\",\n            \"writePointsOk\",\n            \"writeReq\",\n            \"writeReqErr\",\n            \"writeReqOk\"\n          ],\n          \"values\": [\n            [\n              223,\n              0,\n              1,\n              0,\n              0,\n              0,\n              0,\n              0,\n              0,\n              0\n            ]\n          ]\n        },\n        {\n          \"name\": \"tsm1_engine\",\n          \"tags\": {\n            \"database\": \"labview\",\n            \"engine\": \"tsm1\",\n            \"id\": \"20\",\n            \"path\": \"C:\\\\Users\\\\Johan\\\\.influxdb\\\\data\\\\labview\\\\autogen\\\\20\",\n            \"retentionPolicy\": \"autogen\",\n            \"walPath\": \"C:\\\\Users\\\\Johan\\\\.influxdb\\\\wal\\\\labview\\\\autogen\\\\20\"\n          },\n          \"columns\": [\n            \"cacheCompactionDuration\",\n            \"cacheCompactionErr\",\n            \"cacheCompactions\",\n            \"cacheCompactionsActive\",\n            \"tsmFullCompactionDuration\",\n            \"tsmFullCompactionErr\",\n            \"tsmFullCompactionQueue\",\n            \"tsmFullCompactions\",\n            \"tsmFullCompactionsActive\",\n            \"tsmLevel1CompactionDuration\",\n            \"tsmLevel1CompactionErr\",\n            \"tsmLevel1CompactionQueue\",\n            \"tsmLevel1Compactions\",\n            \"tsmLevel1CompactionsActive\",\n            \"tsmLevel2CompactionDuration\",\n            \"tsmLevel2CompactionErr\",\n            \"tsmLevel2CompactionQueue\",\n            \"tsmLevel2Compactions\",\n            \"tsmLevel2CompactionsActive\",\n            \"tsmLevel3CompactionDuration\",\n            \"tsmLevel3CompactionErr\",\n            \"tsmLevel3CompactionQueue\",\n            \"tsmLevel3Compactions\",\n            \"tsmLevel3CompactionsActive\",\n            \"tsmOptimizeCompactionDuration\",\n            \"tsmOptimizeCompactionErr\",\n            \"tsmOptimizeCompactionQueue\",\n            \"tsmOptimizeCompactions\",\n            \"tsmOptimizeCompactionsActive\"\n          ],\n          \"values\": [\n            [\n              0,\n              0,\n              0,\n              0,\n              0,\n              0,\n              0,\n              0,\n              0,\n              0,\n              0,\n              0,\n              0,\n              0,\n              0,\n              0,\n              0,\n              0,\n              0,\n              0,\n              0,\n              0,\n              0,\n              0,\n              0,\n              0,\n              0,\n              0,\n              0\n            ]\n          ]\n        },\n        {\n          \"name\": \"tsm1_cache\",\n          \"tags\": {\n            \"database\": \"labview\",\n            \"engine\": \"tsm1\",\n            \"id\": \"20\",\n            \"path\": \"C:\\\\Users\\\\Johan\\\\.influxdb\\\\data\\\\labview\\\\autogen\\\\20\",\n            \"retentionPolicy\": \"autogen\",\n            \"walPath\": \"C:\\\\Users\\\\Johan\\\\.influxdb\\\\wal\\\\labview\\\\autogen\\\\20\"\n          },\n          \"columns\": [\n            \"WALCompactionTimeMs\",\n            \"cacheAgeMs\",\n            \"cachedBytes\",\n            \"diskBytes\",\n            \"memBytes\",\n            \"snapshotCount\",\n            \"writeDropped\",\n            \"writeErr\",\n            \"writeOk\"\n          ],\n          \"values\": [\n            [\n              0,\n              0,\n              0,\n              0,\n              0,\n              0,\n              0,\n              0,\n              0\n            ]\n          ]\n        },\n        {\n          \"name\": \"tsm1_filestore\",\n          \"tags\": {\n            \"database\": \"labview\",\n            \"engine\": \"tsm1\",\n            \"id\": \"20\",\n            \"path\": \"C:\\\\Users\\\\Johan\\\\.influxdb\\\\data\\\\labview\\\\autogen\\\\20\",\n            \"retentionPolicy\": \"autogen\",\n            \"walPath\": \"C:\\\\Users\\\\Johan\\\\.influxdb\\\\wal\\\\labview\\\\autogen\\\\20\"\n          },\n          \"columns\": [\n            \"diskBytes\",\n            \"numFiles\"\n          ],\n          \"values\": [\n            [\n              223,\n              1\n            ]\n          ]\n        },\n        {\n          \"name\": \"tsm1_wal\",\n          \"tags\": {\n            \"database\": \"labview\",\n            \"engine\": \"tsm1\",\n            \"id\": \"20\",\n            \"path\": \"C:\\\\Users\\\\Johan\\\\.influxdb\\\\data\\\\labview\\\\autogen\\\\20\",\n            \"retentionPolicy\": \"autogen\",\n            \"walPath\": \"C:\\\\Users\\\\Johan\\\\.influxdb\\\\wal\\\\labview\\\\autogen\\\\20\"\n          },\n          \"columns\": [\n            \"currentSegmentDiskBytes\",\n            \"oldSegmentsDiskBytes\",\n            \"writeErr\",\n            \"writeOk\"\n          ],\n          \"values\": [\n            [\n              0,\n              0,\n              0,\n              0\n            ]\n          ]\n        },\n        {\n          \"name\": \"shard\",\n          \"tags\": {\n            \"database\": \"_internal\",\n            \"engine\": \"tsm1\",\n            \"id\": \"21\",\n            \"path\": \"C:\\\\Users\\\\Johan\\\\.influxdb\\\\data\\\\_internal\\\\monitor\\\\21\",\n            \"retentionPolicy\": \"monitor\",\n            \"walPath\": \"C:\\\\Users\\\\Johan\\\\.influxdb\\\\wal\\\\_internal\\\\monitor\\\\21\"\n          },\n          \"columns\": [\n            \"diskBytes\",\n            \"fieldsCreate\",\n            \"seriesCreate\",\n            \"writeBytes\",\n            \"writePointsDropped\",\n            \"writePointsErr\",\n            \"writePointsOk\",\n            \"writeReq\",\n            \"writeReqErr\",\n            \"writeReqOk\"\n          ],\n          \"values\": [\n            [\n              473454,\n              0,\n              109,\n              0,\n              0,\n              0,\n              0,\n              0,\n              0,\n              0\n            ]\n          ]\n        },\n        {\n          \"name\": \"tsm1_engine\",\n          \"tags\": {\n            \"database\": \"_internal\",\n            \"engine\": \"tsm1\",\n            \"id\": \"21\",\n            \"path\": \"C:\\\\Users\\\\Johan\\\\.influxdb\\\\data\\\\_internal\\\\monitor\\\\21\",\n            \"retentionPolicy\": \"monitor\",\n            \"walPath\": \"C:\\\\Users\\\\Johan\\\\.influxdb\\\\wal\\\\_internal\\\\monitor\\\\21\"\n          },\n          \"columns\": [\n            \"cacheCompactionDuration\",\n            \"cacheCompactionErr\",\n            \"cacheCompactions\",\n            \"cacheCompactionsActive\",\n            \"tsmFullCompactionDuration\",\n            \"tsmFullCompactionErr\",\n            \"tsmFullCompactionQueue\",\n            \"tsmFullCompactions\",\n            \"tsmFullCompactionsActive\",\n            \"tsmLevel1CompactionDuration\",\n            \"tsmLevel1CompactionErr\",\n            \"tsmLevel1CompactionQueue\",\n            \"tsmLevel1Compactions\",\n            \"tsmLevel1CompactionsActive\",\n            \"tsmLevel2CompactionDuration\",\n            \"tsmLevel2CompactionErr\",\n            \"tsmLevel2CompactionQueue\",\n            \"tsmLevel2Compactions\",\n            \"tsmLevel2CompactionsActive\",\n            \"tsmLevel3CompactionDuration\",\n            \"tsmLevel3CompactionErr\",\n            \"tsmLevel3CompactionQueue\",\n            \"tsmLevel3Compactions\",\n            \"tsmLevel3CompactionsActive\",\n            \"tsmOptimizeCompactionDuration\",\n            \"tsmOptimizeCompactionErr\",\n            \"tsmOptimizeCompactionQueue\",\n            \"tsmOptimizeCompactions\",\n            \"tsmOptimizeCompactionsActive\"\n          ],\n          \"values\": [\n            [\n              92951500,\n              0,\n              1,\n              0,\n              0,\n              0,\n              0,\n              0,\n              0,\n              0,\n              0,\n              0,\n              0,\n              0,\n              0,\n              0,\n              0,\n              0,\n              0,\n              0,\n              0,\n              0,\n              0,\n              0,\n              0,\n              0,\n              0,\n              0,\n              0\n            ]\n          ]\n        },\n        {\n          \"name\": \"tsm1_cache\",\n          \"tags\": {\n            \"database\": \"_internal\",\n            \"engine\": \"tsm1\",\n            \"id\": \"21\",\n            \"path\": \"C:\\\\Users\\\\Johan\\\\.influxdb\\\\data\\\\_internal\\\\monitor\\\\21\",\n            \"retentionPolicy\": \"monitor\",\n            \"walPath\": \"C:\\\\Users\\\\Johan\\\\.influxdb\\\\wal\\\\_internal\\\\monitor\\\\21\"\n          },\n          \"columns\": [\n            \"WALCompactionTimeMs\",\n            \"cacheAgeMs\",\n            \"cachedBytes\",\n            \"diskBytes\",\n            \"memBytes\",\n            \"snapshotCount\",\n            \"writeDropped\",\n            \"writeErr\",\n            \"writeOk\"\n          ],\n          \"values\": [\n            [\n              92,\n              997,\n              14701786,\n              0,\n              0,\n              0,\n              0,\n              0,\n              1390\n            ]\n          ]\n        },\n        {\n          \"name\": \"tsm1_filestore\",\n          \"tags\": {\n            \"database\": \"_internal\",\n            \"engine\": \"tsm1\",\n            \"id\": \"21\",\n            \"path\": \"C:\\\\Users\\\\Johan\\\\.influxdb\\\\data\\\\_internal\\\\monitor\\\\21\",\n            \"retentionPolicy\": \"monitor\",\n            \"walPath\": \"C:\\\\Users\\\\Johan\\\\.influxdb\\\\wal\\\\_internal\\\\monitor\\\\21\"\n          },\n          \"columns\": [\n            \"diskBytes\",\n            \"numFiles\"\n          ],\n          \"values\": [\n            [\n              473454,\n              1\n            ]\n          ]\n        },\n        {\n          \"name\": \"tsm1_wal\",\n          \"tags\": {\n            \"database\": \"_internal\",\n            \"engine\": \"tsm1\",\n            \"id\": \"21\",\n            \"path\": \"C:\\\\Users\\\\Johan\\\\.influxdb\\\\data\\\\_internal\\\\monitor\\\\21\",\n            \"retentionPolicy\": \"monitor\",\n            \"walPath\": \"C:\\\\Users\\\\Johan\\\\.influxdb\\\\wal\\\\_internal\\\\monitor\\\\21\"\n          },\n          \"columns\": [\n            \"currentSegmentDiskBytes\",\n            \"oldSegmentsDiskBytes\",\n            \"writeErr\",\n            \"writeOk\"\n          ],\n          \"values\": [\n            [\n              0,\n              0,\n              0,\n              0\n            ]\n          ]\n        },\n        {\n          \"name\": \"shard\",\n          \"tags\": {\n            \"database\": \"_internal\",\n            \"engine\": \"tsm1\",\n            \"id\": \"22\",\n            \"path\": \"C:\\\\Users\\\\Johan\\\\.influxdb\\\\data\\\\_internal\\\\monitor\\\\22\",\n            \"retentionPolicy\": \"monitor\",\n            \"walPath\": \"C:\\\\Users\\\\Johan\\\\.influxdb\\\\wal\\\\_internal\\\\monitor\\\\22\"\n          },\n          \"columns\": [\n            \"diskBytes\",\n            \"fieldsCreate\",\n            \"seriesCreate\",\n            \"writeBytes\",\n            \"writePointsDropped\",\n            \"writePointsErr\",\n            \"writePointsOk\",\n            \"writeReq\",\n            \"writeReqErr\",\n            \"writeReqOk\"\n          ],\n          \"values\": [\n            [\n              2344945,\n              655,\n              109,\n              0,\n              0,\n              0,\n              9655,\n              140,\n              0,\n              140\n            ]\n          ]\n        },\n        {\n          \"name\": \"tsm1_engine\",\n          \"tags\": {\n            \"database\": \"_internal\",\n            \"engine\": \"tsm1\",\n            \"id\": \"22\",\n            \"path\": \"C:\\\\Users\\\\Johan\\\\.influxdb\\\\data\\\\_internal\\\\monitor\\\\22\",\n            \"retentionPolicy\": \"monitor\",\n            \"walPath\": \"C:\\\\Users\\\\Johan\\\\.influxdb\\\\wal\\\\_internal\\\\monitor\\\\22\"\n          },\n          \"columns\": [\n            \"cacheCompactionDuration\",\n            \"cacheCompactionErr\",\n            \"cacheCompactions\",\n            \"cacheCompactionsActive\",\n            \"tsmFullCompactionDuration\",\n            \"tsmFullCompactionErr\",\n            \"tsmFullCompactionQueue\",\n            \"tsmFullCompactions\",\n            \"tsmFullCompactionsActive\",\n            \"tsmLevel1CompactionDuration\",\n            \"tsmLevel1CompactionErr\",\n            \"tsmLevel1CompactionQueue\",\n            \"tsmLevel1Compactions\",\n            \"tsmLevel1CompactionsActive\",\n            \"tsmLevel2CompactionDuration\",\n            \"tsmLevel2CompactionErr\",\n            \"tsmLevel2CompactionQueue\",\n            \"tsmLevel2Compactions\",\n            \"tsmLevel2CompactionsActive\",\n            \"tsmLevel3CompactionDuration\",\n            \"tsmLevel3CompactionErr\",\n            \"tsmLevel3CompactionQueue\",\n            \"tsmLevel3Compactions\",\n            \"tsmLevel3CompactionsActive\",\n            \"tsmOptimizeCompactionDuration\",\n            \"tsmOptimizeCompactionErr\",\n            \"tsmOptimizeCompactionQueue\",\n            \"tsmOptimizeCompactions\",\n            \"tsmOptimizeCompactionsActive\"\n          ],\n          \"values\": [\n            [\n              0,\n              0,\n              0,\n              0,\n              0,\n              0,\n              0,\n              0,\n              0,\n              0,\n              0,\n              0,\n              0,\n              0,\n              0,\n              0,\n              0,\n              0,\n              0,\n              0,\n              0,\n              0,\n              0,\n              0,\n              0,\n              0,\n              0,\n              0,\n              0\n            ]\n          ]\n        },\n        {\n          \"name\": \"tsm1_cache\",\n          \"tags\": {\n            \"database\": \"_internal\",\n            \"engine\": \"tsm1\",\n            \"id\": \"22\",\n            \"path\": \"C:\\\\Users\\\\Johan\\\\.influxdb\\\\data\\\\_internal\\\\monitor\\\\22\",\n            \"retentionPolicy\": \"monitor\",\n            \"walPath\": \"C:\\\\Users\\\\Johan\\\\.influxdb\\\\wal\\\\_internal\\\\monitor\\\\22\"\n          },\n          \"columns\": [\n            \"WALCompactionTimeMs\",\n            \"cacheAgeMs\",\n            \"cachedBytes\",\n            \"diskBytes\",\n            \"memBytes\",\n            \"snapshotCount\",\n            \"writeDropped\",\n            \"writeErr\",\n            \"writeOk\"\n          ],\n          \"values\": [\n            [\n              0,\n              1396004,\n              0,\n              0,\n              1735190,\n              0,\n              0,\n              0,\n              140\n            ]\n          ]\n        },\n        {\n          \"name\": \"tsm1_filestore\",\n          \"tags\": {\n            \"database\": \"_internal\",\n            \"engine\": \"tsm1\",\n            \"id\": \"22\",\n            \"path\": \"C:\\\\Users\\\\Johan\\\\.influxdb\\\\data\\\\_internal\\\\monitor\\\\22\",\n            \"retentionPolicy\": \"monitor\",\n            \"walPath\": \"C:\\\\Users\\\\Johan\\\\.influxdb\\\\wal\\\\_internal\\\\monitor\\\\22\"\n          },\n          \"columns\": [\n            \"diskBytes\",\n            \"numFiles\"\n          ],\n          \"values\": [\n            [\n              0,\n              0\n            ]\n          ]\n        },\n        {\n          \"name\": \"tsm1_wal\",\n          \"tags\": {\n            \"database\": \"_internal\",\n            \"engine\": \"tsm1\",\n            \"id\": \"22\",\n            \"path\": \"C:\\\\Users\\\\Johan\\\\.influxdb\\\\data\\\\_internal\\\\monitor\\\\22\",\n            \"retentionPolicy\": \"monitor\",\n            \"walPath\": \"C:\\\\Users\\\\Johan\\\\.influxdb\\\\wal\\\\_internal\\\\monitor\\\\22\"\n          },\n          \"columns\": [\n            \"currentSegmentDiskBytes\",\n            \"oldSegmentsDiskBytes\",\n            \"writeErr\",\n            \"writeOk\"\n          ],\n          \"values\": [\n            [\n              2344945,\n              0,\n              0,\n              140\n            ]\n          ]\n        },\n        {\n          \"name\": \"write\",\n          \"columns\": [\n            \"pointReq\",\n            \"pointReqLocal\",\n            \"req\",\n            \"subWriteDrop\",\n            \"subWriteOk\",\n            \"writeDrop\",\n            \"writeError\",\n            \"writeOk\",\n            \"writeTimeout\"\n          ],\n          \"values\": [\n            [\n              9655,\n              9655,\n              140,\n              0,\n              140,\n              0,\n              0,\n              140,\n              0\n            ]\n          ]\n        },\n        {\n          \"name\": \"subscriber\",\n          \"columns\": [\n            \"createFailures\",\n            \"pointsWritten\",\n            \"writeFailures\"\n          ],\n          \"values\": [\n            [\n              0,\n              0,\n              0\n            ]\n          ]\n        },\n        {\n          \"name\": \"cq\",\n          \"columns\": [\n            \"queryFail\",\n            \"queryOk\"\n          ],\n          \"values\": [\n            [\n              0,\n              0\n            ]\n          ]\n        },\n        {\n          \"name\": \"httpd\",\n          \"tags\": {\n            \"bind\": \":8086\"\n          },\n          \"columns\": [\n            \"authFail\",\n            \"clientError\",\n            \"pingReq\",\n            \"pointsWrittenDropped\",\n            \"pointsWrittenFail\",\n            \"pointsWrittenOK\",\n            \"promReadReq\",\n            \"promWriteReq\",\n            \"queryReq\",\n            \"queryReqDurationNs\",\n            \"queryRespBytes\",\n            \"recoveredPanics\",\n            \"req\",\n            \"reqActive\",\n            \"reqDurationNs\",\n            \"serverError\",\n            \"statusReq\",\n            \"writeReq\",\n            \"writeReqActive\",\n            \"writeReqBytes\",\n            \"writeReqDurationNs\"\n          ],\n          \"values\": [\n            [\n              0,\n              1,\n              0,\n              0,\n              0,\n              0,\n              0,\n              0,\n              11,\n              86995000,\n              908,\n              0,\n              11,\n              1,\n              108000400,\n              0,\n              0,\n              0,\n              0,\n              0,\n              0\n            ]\n          ]\n        }\n      ]\n    }\n  ]\n}"
  (unwired) string[] ["{\n  \"results\": [\n    {\n      \"statement_id\": 0,\n      \"error\": \"database not found: InvalidDB\"\n    }\n  ]\n}", "{\n  \"results\": [\n    {\n      \"statement_id\": 0\n    }\n  ]\n}", "{\n  \"results\": [\n    {\n      \"statement_id\": 0,\n      \"series\": [\n        {\n          \"name\": \"databases\",\n          \"columns\": [\n            \"name\"\n          ],\n          \"values\": [\n            [\n              \"_internal\"\n            ],\n            [\n              \"data\"\n            ],\n            [\n              \"labview\"\n            ]\n          ]\n        }\n      ]\n    }\n  ]\n}", "{\n  \"results\": [\n    {\n      \"statement_id\": 0,\n      \"series\": [\n        {\n          \"name\": \"mymeas\",\n          \"columns\": [\n            \"time\",\n            \"myfield\",\n            \"mytag1\",\n            \"mytag2\"\n          ],\n          \"values\": [\n            [\n              \"2017-03-01T00:16:18Z\",\n              33.1,\n              null,\n              null\n            ],\n            [\n              \"2017-03-01T00:17:18Z\",\n              12.4,\n              \"12\",\n              \"14\"\n            ]\n          ]\n        }\n      ]\n    }\n  ]\n}", "{\n  \"results\": [\n    {\n      \"statement_id\": 0,\n      \"series\": [\n        {\n          \"columns\": [\n            \"name\",\n            \"duration\",\n            \"shardGroupDuration\",\n            \"replicaN\",\n            \"default\"\n          ],\n          \"values\": [\n            [\n              \"autogen\",\n              \"0s\",\n              \"168h0m0s\",\n              1,\n              true\n            ]\n          ]\n        }\n      ]\n    }\n  ]\n}", "{\n  \"results\": [\n    {\n      \"statement_id\": 0,\n      \"series\": [\n        {\n          \"name\": \"_internal\",\n          \"columns\": [\n            \"name\",\n            \"query\"\n          ]\n        },\n        {\n          \"name\": \"data\",\n          \"columns\": [\n            \"name\",\n            \"query\"\n          ]\n        },\n        {\n          \"name\": \"labview\",\n          \"columns\": [\n            \"name\",\n            \"query\"\n          ]\n        },\n        {\n          \"name\": \"testDB\",\n          \"columns\": [\n            \"name\",\n            \"query\"\n          ],\n          \"values\": [\n            [\n              \"TestCQ\",\n              \"CREATE CONTINUOUS QUERY TestCQ ON testDB BEGIN SELECT mean(Doublefield) AS Doublefield INTO testDB.autogen.cqMeasurement FROM testDB.autogen.TestMeasurement GROUP BY time(1h), * END\"\n            ],\n            [\n              \"TestCQ1\",\n              \"CREATE CONTINUOUS QUERY TestCQ1 ON testDB RESAMPLE EVERY 30m FOR 2h BEGIN SELECT mean(Intfield) AS Intfield INTO testDB.autogen.cqMeasurement FROM testDB.autogen.TestMeasurement GROUP BY time(1h), * END\"\n            ]\n          ]\n        }\n      ]\n    }\n  ]\n}", "{\n  \"results\": [\n    {\n      \"statement_id\": 0,\n      \"series\": [\n        {\n          \"name\": \"runtime\",\n          \"columns\": [\n            \"Alloc\",\n            \"Frees\",\n            \"HeapAlloc\",\n            \"HeapIdle\",\n            \"HeapInUse\",\n            \"HeapObjects\",\n            \"HeapReleased\",\n            \"HeapSys\",\n            \"Lookups\",\n            \"Mallocs\",\n            \"NumGC\",\n            \"NumGoroutine\",\n            \"PauseTotalNs\",\n            \"Sys\",\n            \"TotalAlloc\"\n          ],\n          \"values\": [\n            [\n              10031728,\n              4491960,\n              10031728,\n              68689920,\n              12771328,\n              133250,\n              59473920,\n              81461248,\n              269,\n              4625210,\n              73,\n              27,\n              4009300,\n              89569528,\n              888359040\n            ]\n          ]\n        },\n        {\n          \"name\": \"queryExecutor\",\n          \"columns\": [\n            \"queriesActive\",\n            \"queriesExecuted\",\n            \"queriesFinished\",\n            \"queryDurationNs\",\n            \"recoveredPanics\"\n          ],\n          \"values\": [\n            [\n              1,\n              10,\n              9,\n              64001100,\n              0\n            ]\n          ]\n        },\n        {\n          \"name\": \"database\",\n          \"tags\": {\n            \"database\": \"_internal\"\n          },\n          \"columns\": [\n            \"numMeasurements\",\n            \"numSeries\"\n          ],\n          \"values\": [\n            [\n              12,\n              108\n            ]\n          ]\n        },\n        {\n          \"name\": \"database\",\n          \"tags\": {\n            \"database\": \"labview\"\n          },\n          \"columns\": [\n            \"numMeasurements\",\n            \"numSeries\"\n          ],\n          \"values\": [\n            [\n              1,\n              1\n            ]\n          ]\n        },\n        {\n          \"name\": \"database\",\n          \"tags\": {\n            \"database\": \"data\"\n          },\n          \"columns\": [\n            \"numMeasurements\",\n            \"numSeries\"\n          ],\n          \"values\": [\n            [\n              7,\n              23\n            ]\n          ]\n        },\n        {\n          \"name\": \"shard\",\n          \"tags\": {\n            \"database\": \"_internal\",\n            \"engine\": \"tsm1\",\n            \"id\": \"6\",\n            \"path\": \"C:\\\\Users\\\\Johan\\\\.influxdb\\\\data\\\\_internal\\\\monitor\\\\6\",\n            \"retentionPolicy\": \"monitor\",\n            \"walPath\": \"C:\\\\Users\\\\Johan\\\\.influxdb\\\\wal\\\\_internal\\\\monitor\\\\6\"\n          },\n          \"columns\": [\n            \"diskBytes\",\n            \"fieldsCreate\",\n            \"seriesCreate\",\n            \"writeBytes\",\n            \"writePointsDropped\",\n            \"writePointsErr\",\n            \"writePointsOk\",\n            \"writeReq\",\n            \"writeReqErr\",\n            \"writeReqOk\"\n          ],\n          \"values\": [\n            [\n              260046,\n              0,\n              109,\n              0,\n              0,\n              0,\n              0,\n              0,\n              0,\n              0\n            ]\n          ]\n        },\n        {\n          \"name\": \"tsm1_engine\",\n          \"tags\": {\n            \"database\": \"_internal\",\n            \"engine\": \"tsm1\",\n            \"id\": \"6\",\n            \"path\": \"C:\\\\Users\\\\Johan\\\\.influxdb\\\\data\\\\_internal\\\\monitor\\\\6\",\n            \"retentionPolicy\": \"monitor\",\n            \"walPath\": \"C:\\\\Users\\\\Johan\\\\.influxdb\\\\wal\\\\_internal\\\\monitor\\\\6\"\n          },\n          \"columns\": [\n            \"cacheCompactionDuration\",\n            \"cacheCompactionErr\",\n            \"cacheCompactions\",\n            \"cacheCompactionsActive\",\n            \"tsmFullCompactionDuration\",\n            \"tsmFullCompactionErr\",\n            \"tsmFullCompactionQueue\",\n            \"tsmFullCompactions\",\n            \"tsmFullCompactionsActive\",\n            \"tsmLevel1CompactionDuration\",\n            \"tsmLevel1CompactionErr\",\n            \"tsmLevel1CompactionQueue\",\n            \"tsmLevel1Compactions\",\n            \"tsmLevel1CompactionsActive\",\n            \"tsmLevel2CompactionDuration\",\n            \"tsmLevel2CompactionErr\",\n            \"tsmLevel2CompactionQueue\",\n            \"tsmLevel2Compactions\",\n            \"tsmLevel2CompactionsActive\",\n            \"tsmLevel3CompactionDuration\",\n            \"tsmLevel3CompactionErr\",\n            \"tsmLevel3CompactionQueue\",\n            \"tsmLevel3Compactions\",\n            \"tsmLevel3CompactionsActive\",\n            \"tsmOptimizeCompactionDuration\",\n            \"tsmOptimizeCompactionErr\",\n            \"tsmOptimizeCompactionQueue\",\n            \"tsmOptimizeCompactions\",\n            \"tsmOptimizeCompactionsActive\"\n          ],\n          \"values\": [\n            [\n              0,\n              0,\n              0,\n              0,\n              0,\n              0,\n              0,\n              0,\n              0,\n              0,\n              0,\n              0,\n              0,\n              0,\n              0,\n              0,\n              0,\n              0,\n              0,\n              0,\n              0,\n              0,\n              0,\n              0,\n              0,\n              0,\n              0,\n              0,\n              0\n            ]\n          ]\n        },\n        {\n          \"name\": \"tsm1_cache\",\n          \"tags\": {\n            \"database\": \"_internal\",\n            \"engine\": \"tsm1\",\n            \"id\": \"6\",\n            \"path\": \"C:\\\\Users\\\\Johan\\\\.influxdb\\\\data\\\\_internal\\\\monitor\\\\6\",\n            \"retentionPolicy\": \"monitor\",\n            \"walPath\": \"C:\\\\Users\\\\Johan\\\\.influxdb\\\\wal\\\\_internal\\\\monitor\\\\6\"\n          },\n          \"columns\": [\n            \"WALCompactionTimeMs\",\n            \"cacheAgeMs\",\n            \"cachedBytes\",\n            \"diskBytes\",\n            \"memBytes\",\n            \"snapshotCount\",\n            \"writeDropped\",\n            \"writeErr\",\n            \"writeOk\"\n          ],\n          \"values\": [\n            [\n              0,\n              0,\n              0,\n              0,\n              0,\n              0,\n              0,\n              0,\n              0\n            ]\n          ]\n        },\n        {\n          \"name\": \"tsm1_filestore\",\n          \"tags\": {\n            \"database\": \"_internal\",\n            \"engine\": \"tsm1\",\n            \"id\": \"6\",\n            \"path\": \"C:\\\\Users\\\\Johan\\\\.influxdb\\\\data\\\\_internal\\\\monitor\\\\6\",\n            \"retentionPolicy\": \"monitor\",\n            \"walPath\": \"C:\\\\Users\\\\Johan\\\\.influxdb\\\\wal\\\\_internal\\\\monitor\\\\6\"\n          },\n          \"columns\": [\n            \"diskBytes\",\n            \"numFiles\"\n          ],\n          \"values\": [\n            [\n              260046,\n              1\n            ]\n          ]\n        },\n        {\n          \"name\": \"tsm1_wal\",\n          \"tags\": {\n            \"database\": \"_internal\",\n            \"engine\": \"tsm1\",\n            \"id\": \"6\",\n            \"path\": \"C:\\\\Users\\\\Johan\\\\.influxdb\\\\data\\\\_internal\\\\monitor\\\\6\",\n            \"retentionPolicy\": \"monitor\",\n            \"walPath\": \"C:\\\\Users\\\\Johan\\\\.influxdb\\\\wal\\\\_internal\\\\monitor\\\\6\"\n          },\n          \"columns\": [\n            \"currentSegmentDiskBytes\",\n            \"oldSegmentsDiskBytes\",\n            \"writeErr\",\n            \"writeOk\"\n          ],\n          \"values\": [\n            [\n              0,\n              0,\n              0,\n              0\n            ]\n          ]\n        },\n        {\n          \"name\": \"shard\",\n          \"tags\": {\n            \"database\": \"data\",\n            \"engine\": \"tsm1\",\n            \"id\": \"10\",\n            \"path\": \"C:\\\\Users\\\\Johan\\\\.influxdb\\\\data\\\\data\\\\autogen\\\\10\",\n            \"retentionPolicy\": \"autogen\",\n            \"walPath\": \"C:\\\\Users\\\\Johan\\\\.influxdb\\\\wal\\\\data\\\\autogen\\\\10\"\n          },\n          \"columns\": [\n            \"diskBytes\",\n            \"fieldsCreate\",\n            \"seriesCreate\",\n            \"writeBytes\",\n            \"writePointsDropped\",\n            \"writePointsErr\",\n            \"writePointsOk\",\n            \"writeReq\",\n            \"writeReqErr\",\n            \"writeReqOk\"\n          ],\n          \"values\": [\n            [\n              614,\n              0,\n              23,\n              0,\n              0,\n              0,\n              0,\n              0,\n              0,\n              0\n            ]\n          ]\n        },\n        {\n          \"name\": \"tsm1_engine\",\n          \"tags\": {\n            \"database\": \"data\",\n            \"engine\": \"tsm1\",\n            \"id\": \"10\",\n            \"path\": \"C:\\\\Users\\\\Johan\\\\.influxdb\\\\data\\\\data\\\\autogen\\\\10\",\n            \"retentionPolicy\": \"autogen\",\n            \"walPath\": \"C:\\\\Users\\\\Johan\\\\.influxdb\\\\wal\\\\data\\\\autogen\\\\10\"\n          },\n          \"columns\": [\n            \"cacheCompactionDuration\",\n            \"cacheCompactionErr\",\n            \"cacheCompactions\",\n            \"cacheCompactionsActive\",\n            \"tsmFullCompactionDuration\",\n            \"tsmFullCompactionErr\",\n            \"tsmFullCompactionQueue\",\n            \"tsmFullCompactions\",\n            \"tsmFullCompactionsActive\",\n            \"tsmLevel1CompactionDuration\",\n            \"tsmLevel1CompactionErr\",\n            \"tsmLevel1CompactionQueue\",\n            \"tsmLevel1Compactions\",\n            \"tsmLevel1CompactionsActive\",\n            \"tsmLevel2CompactionDuration\",\n            \"tsmLevel2CompactionErr\",\n            \"tsmLevel2CompactionQueue\",\n            \"tsmLevel2Compactions\",\n            \"tsmLevel2CompactionsActive\",\n            \"tsmLevel3CompactionDuration\",\n            \"tsmLevel3CompactionErr\",\n            \"tsmLevel3CompactionQueue\",\n            \"tsmLevel3Compactions\",\n            \"tsmLevel3CompactionsActive\",\n            \"tsmOptimizeCompactionDuration\",\n            \"tsmOptimizeCompactionErr\",\n            \"tsmOptimizeCompactionQueue\",\n            \"tsmOptimizeCompactions\",\n            \"tsmOptimizeCompactionsActive\"\n          ],\n          \"values\": [\n            [\n              0,\n              0,\n              0,\n              0,\n              0,\n              0,\n              0,\n              0,\n              0,\n              0,\n              0,\n              0,\n              0,\n              0,\n              0,\n              0,\n              0,\n              0,\n              0,\n              0,\n              0,\n              0,\n              0,\n              0,\n              0,\n              0,\n              0,\n              0,\n              0\n            ]\n          ]\n        },\n        {\n          \"name\": \"tsm1_cache\",\n          \"tags\": {\n            \"database\": \"data\",\n            \"engine\": \"tsm1\",\n            \"id\": \"10\",\n            \"path\": \"C:\\\\Users\\\\Johan\\\\.influxdb\\\\data\\\\data\\\\autogen\\\\10\",\n            \"retentionPolicy\": \"autogen\",\n            \"walPath\": \"C:\\\\Users\\\\Johan\\\\.influxdb\\\\wal\\\\data\\\\autogen\\\\10\"\n          },\n          \"columns\": [\n            \"WALCompactionTimeMs\",\n            \"cacheAgeMs\",\n            \"cachedBytes\",\n            \"diskBytes\",\n            \"memBytes\",\n            \"snapshotCount\",\n            \"writeDropped\",\n            \"writeErr\",\n            \"writeOk\"\n          ],\n          \"values\": [\n            [\n              0,\n              0,\n              0,\n              0,\n              0,\n              0,\n              0,\n              0,\n              0\n            ]\n          ]\n        },\n        {\n          \"name\": \"tsm1_filestore\",\n          \"tags\": {\n            \"database\": \"data\",\n            \"engine\": \"tsm1\",\n            \"id\": \"10\",\n            \"path\": \"C:\\\\Users\\\\Johan\\\\.influxdb\\\\data\\\\data\\\\autogen\\\\10\",\n            \"retentionPolicy\": \"autogen\",\n            \"walPath\": \"C:\\\\Users\\\\Johan\\\\.influxdb\\\\wal\\\\data\\\\autogen\\\\10\"\n          },\n          \"columns\": [\n            \"diskBytes\",\n            \"numFiles\"\n          ],\n          \"values\": [\n            [\n              614,\n              1\n            ]\n          ]\n        },\n        {\n          \"name\": \"tsm1_wal\",\n          \"tags\": {\n            \"database\": \"data\",\n            \"engine\": \"tsm1\",\n            \"id\": \"10\",\n            \"path\": \"C:\\\\Users\\\\Johan\\\\.influxdb\\\\data\\\\data\\\\autogen\\\\10\",\n            \"retentionPolicy\": \"autogen\",\n            \"walPath\": \"C:\\\\Users\\\\Johan\\\\.influxdb\\\\wal\\\\data\\\\autogen\\\\10\"\n          },\n          \"columns\": [\n            \"currentSegmentDiskBytes\",\n            \"oldSegmentsDiskBytes\",\n            \"writeErr\",\n            \"writeOk\"\n          ],\n          \"values\": [\n            [\n              0,\n              0,\n              0,\n              0\n            ]\n          ]\n        },\n        {\n          \"name\": \"shard\",\n          \"tags\": {\n            \"database\": \"data\",\n            \"engine\": \"tsm1\",\n            \"id\": \"11\",\n            \"path\": \"C:\\\\Users\\\\Johan\\\\.influxdb\\\\data\\\\data\\\\autogen\\\\11\",\n            \"retentionPolicy\": \"autogen\",\n            \"walPath\": \"C:\\\\Users\\\\Johan\\\\.influxdb\\\\wal\\\\data\\\\autogen\\\\11\"\n          },\n          \"columns\": [\n            \"diskBytes\",\n            \"fieldsCreate\",\n            \"seriesCreate\",\n            \"writeBytes\",\n            \"writePointsDropped\",\n            \"writePointsErr\",\n            \"writePointsOk\",\n            \"writeReq\",\n            \"writeReqErr\",\n            \"writeReqOk\"\n          ],\n          \"values\": [\n            [\n              115,\n              0,\n              23,\n              0,\n              0,\n              0,\n              0,\n              0,\n              0,\n              0\n            ]\n          ]\n        },\n        {\n          \"name\": \"tsm1_engine\",\n          \"tags\": {\n            \"database\": \"data\",\n            \"engine\": \"tsm1\",\n            \"id\": \"11\",\n            \"path\": \"C:\\\\Users\\\\Johan\\\\.influxdb\\\\data\\\\data\\\\autogen\\\\11\",\n            \"retentionPolicy\": \"autogen\",\n            \"walPath\": \"C:\\\\Users\\\\Johan\\\\.influxdb\\\\wal\\\\data\\\\autogen\\\\11\"\n          },\n          \"columns\": [\n            \"cacheCompactionDuration\",\n            \"cacheCompactionErr\",\n            \"cacheCompactions\",\n            \"cacheCompactionsActive\",\n            \"tsmFullCompactionDuration\",\n            \"tsmFullCompactionErr\",\n            \"tsmFullCompactionQueue\",\n            \"tsmFullCompactions\",\n            \"tsmFullCompactionsActive\",\n            \"tsmLevel1CompactionDuration\",\n            \"tsmLevel1CompactionErr\",\n            \"tsmLevel1CompactionQueue\",\n            \"tsmLevel1Compactions\",\n            \"tsmLevel1CompactionsActive\",\n            \"tsmLevel2CompactionDuration\",\n            \"tsmLevel2CompactionErr\",\n            \"tsmLevel2CompactionQueue\",\n            \"tsmLevel2Compactions\",\n            \"tsmLevel2CompactionsActive\",\n            \"tsmLevel3CompactionDuration\",\n            \"tsmLevel3CompactionErr\",\n            \"tsmLevel3CompactionQueue\",\n            \"tsmLevel3Compactions\",\n            \"tsmLevel3CompactionsActive\",\n            \"tsmOptimizeCompactionDuration\",\n            \"tsmOptimizeCompactionErr\",\n            \"tsmOptimizeCompactionQueue\",\n            \"tsmOptimizeCompactions\",\n            \"tsmOptimizeCompactionsActive\"\n          ],\n          \"values\": [\n            [\n              0,\n              0,\n              0,\n              0,\n              0,\n              0,\n              0,\n              0,\n              0,\n              0,\n              0,\n              0,\n              0,\n              0,\n              0,\n              0,\n              0,\n              0,\n              0,\n              0,\n              0,\n              0,\n              0,\n              0,\n              0,\n              0,\n              0,\n              0,\n              0\n            ]\n          ]\n        },\n        {\n          \"name\": \"tsm1_cache\",\n          \"tags\": {\n            \"database\": \"data\",\n            \"engine\": \"tsm1\",\n            \"id\": \"11\",\n            \"path\": \"C:\\\\Users\\\\Johan\\\\.influxdb\\\\data\\\\data\\\\autogen\\\\11\",\n            \"retentionPolicy\": \"autogen\",\n            \"walPath\": \"C:\\\\Users\\\\Johan\\\\.influxdb\\\\wal\\\\data\\\\autogen\\\\11\"\n          },\n          \"columns\": [\n            \"WALCompactionTimeMs\",\n            \"cacheAgeMs\",\n            \"cachedBytes\",\n            \"diskBytes\",\n            \"memBytes\",\n            \"snapshotCount\",\n            \"writeDropped\",\n            \"writeErr\",\n            \"writeOk\"\n          ],\n          \"values\": [\n            [\n              0,\n              0,\n              0,\n              0,\n              0,\n              0,\n              0,\n              0,\n              0\n            ]\n          ]\n        },\n        {\n          \"name\": \"tsm1_filestore\",\n          \"tags\": {\n            \"database\": \"data\",\n            \"engine\": \"tsm1\",\n            \"id\": \"11\",\n            \"path\": \"C:\\\\Users\\\\Johan\\\\.influxdb\\\\data\\\\data\\\\autogen\\\\11\",\n            \"retentionPolicy\": \"autogen\",\n            \"walPath\": \"C:\\\\Users\\\\Johan\\\\.influxdb\\\\wal\\\\data\\\\autogen\\\\11\"\n          },\n          \"columns\": [\n            \"diskBytes\",\n            \"numFiles\"\n          ],\n          \"values\": [\n            [\n              115,\n              1\n            ]\n          ]\n        },\n        {\n          \"name\": \"tsm1_wal\",\n          \"tags\": {\n            \"database\": \"data\",\n            \"engine\": \"tsm1\",\n            \"id\": \"11\",\n            \"path\": \"C:\\\\Users\\\\Johan\\\\.influxdb\\\\data\\\\data\\\\autogen\\\\11\",\n            \"retentionPolicy\": \"autogen\",\n            \"walPath\": \"C:\\\\Users\\\\Johan\\\\.influxdb\\\\wal\\\\data\\\\autogen\\\\11\"\n          },\n          \"columns\": [\n            \"currentSegmentDiskBytes\",\n            \"oldSegmentsDiskBytes\",\n            \"writeErr\",\n            \"writeOk\"\n          ],\n          \"values\": [\n            [\n              0,\n              0,\n              0,\n              0\n            ]\n          ]\n        },\n        {\n          \"name\": \"shard\",\n          \"tags\": {\n            \"database\": \"data\",\n            \"engine\": \"tsm1\",\n            \"id\": \"12\",\n            \"path\": \"C:\\\\Users\\\\Johan\\\\.influxdb\\\\data\\\\data\\\\autogen\\\\12\",\n            \"retentionPolicy\": \"autogen\",\n            \"walPath\": \"C:\\\\Users\\\\Johan\\\\.influxdb\\\\wal\\\\data\\\\autogen\\\\12\"\n          },\n          \"columns\": [\n            \"diskBytes\",\n            \"fieldsCreate\",\n            \"seriesCreate\",\n            \"writeBytes\",\n            \"writePointsDropped\",\n            \"writePointsErr\",\n            \"writePointsOk\",\n            \"writeReq\",\n            \"writeReqErr\",\n            \"writeReqOk\"\n          ],\n          \"values\": [\n            [\n              58924,\n              0,\n              23,\n              0,\n              0,\n              0,\n              0,\n              0,\n              0,\n              0\n            ]\n          ]\n        },\n        {\n          \"name\": \"tsm1_engine\",\n          \"tags\": {\n            \"database\": \"data\",\n            \"engine\": \"tsm1\",\n            \"id\": \"12\",\n            \"path\": \"C:\\\\Users\\\\Johan\\\\.influxdb\\\\data\\\\data\\\\autogen\\\\12\",\n            \"retentionPolicy\": \"autogen\",\n            \"walPath\": \"C:\\\\Users\\\\Johan\\\\.influxdb\\\\wal\\\\data\\\\autogen\\\\12\"\n          },\n          \"columns\": [\n            \"cacheCompactionDuration\",\n            \"cacheCompactionErr\",\n            \"cacheCompactions\",\n            \"cacheCompactionsActive\",\n            \"tsmFullCompactionDuration\",\n            \"tsmFullCompactionErr\",\n            \"tsmFullCompactionQueue\",\n            \"tsmFullCompactions\",\n            \"tsmFullCompactionsActive\",\n            \"tsmLevel1CompactionDuration\",\n            \"tsmLevel1CompactionErr\",\n            \"tsmLevel1CompactionQueue\",\n            \"tsmLevel1Compactions\",\n            \"tsmLevel1CompactionsActive\",\n            \"tsmLevel2CompactionDuration\",\n            \"tsmLevel2CompactionErr\",\n            \"tsmLevel2CompactionQueue\",\n            \"tsmLevel2Compactions\",\n            \"tsmLevel2CompactionsActive\",\n            \"tsmLevel3CompactionDuration\",\n            \"tsmLevel3CompactionErr\",\n            \"tsmLevel3CompactionQueue\",\n            \"tsmLevel3Compactions\",\n            \"tsmLevel3CompactionsActive\",\n            \"tsmOptimizeCompactionDuration\",\n            \"tsmOptimizeCompactionErr\",\n            \"tsmOptimizeCompactionQueue\",\n            \"tsmOptimizeCompactions\",\n            \"tsmOptimizeCompactionsActive\"\n          ],\n          \"values\": [\n            [\n              0,\n              0,\n              0,\n              0,\n              0,\n              0,\n              0,\n              0,\n              0,\n              0,\n              0,\n              0,\n              0,\n              0,\n              0,\n              0,\n              0,\n              0,\n              0,\n              0,\n              0,\n              0,\n              0,\n              0,\n              0,\n              0,\n              0,\n              0,\n              0\n            ]\n          ]\n        },\n        {\n          \"name\": \"tsm1_cache\",\n          \"tags\": {\n            \"database\": \"data\",\n            \"engine\": \"tsm1\",\n            \"id\": \"12\",\n            \"path\": \"C:\\\\Users\\\\Johan\\\\.influxdb\\\\data\\\\data\\\\autogen\\\\12\",\n            \"retentionPolicy\": \"autogen\",\n            \"walPath\": \"C:\\\\Users\\\\Johan\\\\.influxdb\\\\wal\\\\data\\\\autogen\\\\12\"\n          },\n          \"columns\": [\n            \"WALCompactionTimeMs\",\n            \"cacheAgeMs\",\n            \"cachedBytes\",\n            \"diskBytes\",\n            \"memBytes\",\n            \"snapshotCount\",\n            \"writeDropped\",\n            \"writeErr\",\n            \"writeOk\"\n          ],\n          \"values\": [\n            [\n              0,\n              0,\n              0,\n              0,\n              0,\n              0,\n              0,\n              0,\n              0\n            ]\n          ]\n        },\n        {\n          \"name\": \"tsm1_filestore\",\n          \"tags\": {\n            \"database\": \"data\",\n            \"engine\": \"tsm1\",\n            \"id\": \"12\",\n            \"path\": \"C:\\\\Users\\\\Johan\\\\.influxdb\\\\data\\\\data\\\\autogen\\\\12\",\n            \"retentionPolicy\": \"autogen\",\n            \"walPath\": \"C:\\\\Users\\\\Johan\\\\.influxdb\\\\wal\\\\data\\\\autogen\\\\12\"\n          },\n          \"columns\": [\n            \"diskBytes\",\n            \"numFiles\"\n          ],\n          \"values\": [\n            [\n              58924,\n              1\n            ]\n          ]\n        },\n        {\n          \"name\": \"tsm1_wal\",\n          \"tags\": {\n            \"database\": \"data\",\n            \"engine\": \"tsm1\",\n            \"id\": \"12\",\n            \"path\": \"C:\\\\Users\\\\Johan\\\\.influxdb\\\\data\\\\data\\\\autogen\\\\12\",\n            \"retentionPolicy\": \"autogen\",\n            \"walPath\": \"C:\\\\Users\\\\Johan\\\\.influxdb\\\\wal\\\\data\\\\autogen\\\\12\"\n          },\n          \"columns\": [\n            \"currentSegmentDiskBytes\",\n            \"oldSegmentsDiskBytes\",\n            \"writeErr\",\n            \"writeOk\"\n          ],\n          \"values\": [\n            [\n              0,\n              0,\n              0,\n              0\n            ]\n          ]\n        },\n        {\n          \"name\": \"shard\",\n          \"tags\": {\n            \"database\": \"_internal\",\n            \"engine\": \"tsm1\",\n            \"id\": \"13\",\n            \"path\": \"C:\\\\Users\\\\Johan\\\\.influxdb\\\\data\\\\_internal\\\\monitor\\\\13\",\n            \"retentionPolicy\": \"monitor\",\n            \"walPath\": \"C:\\\\Users\\\\Johan\\\\.influxdb\\\\wal\\\\_internal\\\\monitor\\\\13\"\n          },\n          \"columns\": [\n            \"diskBytes\",\n            \"fieldsCreate\",\n            \"seriesCreate\",\n            \"writeBytes\",\n            \"writePointsDropped\",\n            \"writePointsErr\",\n            \"writePointsOk\",\n            \"writeReq\",\n            \"writeReqErr\",\n            \"writeReqOk\"\n          ],\n          \"values\": [\n            [\n              157086,\n              0,\n              109,\n              0,\n              0,\n              0,\n              0,\n              0,\n              0,\n              0\n            ]\n          ]\n        },\n        {\n          \"name\": \"tsm1_engine\",\n          \"tags\": {\n            \"database\": \"_internal\",\n            \"engine\": \"tsm1\",\n            \"id\": \"13\",\n            \"path\": \"C:\\\\Users\\\\Johan\\\\.influxdb\\\\data\\\\_internal\\\\monitor\\\\13\",\n            \"retentionPolicy\": \"monitor\",\n            \"walPath\": \"C:\\\\Users\\\\Johan\\\\.influxdb\\\\wal\\\\_internal\\\\monitor\\\\13\"\n          },\n          \"columns\": [\n            \"cacheCompactionDuration\",\n            \"cacheCompactionErr\",\n            \"cacheCompactions\",\n            \"cacheCompactionsActive\",\n            \"tsmFullCompactionDuration\",\n            \"tsmFullCompactionErr\",\n            \"tsmFullCompactionQueue\",\n            \"tsmFullCompactions\",\n            \"tsmFullCompactionsActive\",\n            \"tsmLevel1CompactionDuration\",\n            \"tsmLevel1CompactionErr\",\n            \"tsmLevel1CompactionQueue\",\n            \"tsmLevel1Compactions\",\n            \"tsmLevel1CompactionsActive\",\n            \"tsmLevel2CompactionDuration\",\n            \"tsmLevel2CompactionErr\",\n            \"tsmLevel2CompactionQueue\",\n            \"tsmLevel2Compactions\",\n            \"tsmLevel2CompactionsActive\",\n            \"tsmLevel3CompactionDuration\",\n            \"tsmLevel3CompactionErr\",\n            \"tsmLevel3CompactionQueue\",\n            \"tsmLevel3Compactions\",\n            \"tsmLevel3CompactionsActive\",\n            \"tsmOptimizeCompactionDuration\",\n            \"tsmOptimizeCompactionErr\",\n            \"tsmOptimizeCompactionQueue\",\n            \"tsmOptimizeCompactions\",\n            \"tsmOptimizeCompactionsActive\"\n          ],\n          \"values\": [\n            [\n              0,\n              0,\n              0,\n              0,\n              0,\n              0,\n              0,\n              0,\n              0,\n              0,\n              0,\n              0,\n              0,\n              0,\n              0,\n              0,\n              0,\n              0,\n              0,\n              0,\n              0,\n              0,\n              0,\n              0,\n              0,\n              0,\n              0,\n              0,\n              0\n            ]\n          ]\n        },\n        {\n          \"name\": \"tsm1_cache\",\n          \"tags\": {\n            \"database\": \"_internal\",\n            \"engine\": \"tsm1\",\n            \"id\": \"13\",\n            \"path\": \"C:\\\\Users\\\\Johan\\\\.influxdb\\\\data\\\\_internal\\\\monitor\\\\13\",\n            \"retentionPolicy\": \"monitor\",\n            \"walPath\": \"C:\\\\Users\\\\Johan\\\\.influxdb\\\\wal\\\\_internal\\\\monitor\\\\13\"\n          },\n          \"columns\": [\n            \"WALCompactionTimeMs\",\n            \"cacheAgeMs\",\n            \"cachedBytes\",\n            \"diskBytes\",\n            \"memBytes\",\n            \"snapshotCount\",\n            \"writeDropped\",\n            \"writeErr\",\n            \"writeOk\"\n          ],\n          \"values\": [\n            [\n              0,\n              0,\n              0,\n              0,\n              0,\n              0,\n              0,\n              0,\n              0\n            ]\n          ]\n        },\n        {\n          \"name\": \"tsm1_filestore\",\n          \"tags\": {\n            \"database\": \"_internal\",\n            \"engine\": \"tsm1\",\n            \"id\": \"13\",\n            \"path\": \"C:\\\\Users\\\\Johan\\\\.influxdb\\\\data\\\\_internal\\\\monitor\\\\13\",\n            \"retentionPolicy\": \"monitor\",\n            \"walPath\": \"C:\\\\Users\\\\Johan\\\\.influxdb\\\\wal\\\\_internal\\\\monitor\\\\13\"\n          },\n          \"columns\": [\n            \"diskBytes\",\n            \"numFiles\"\n          ],\n          \"values\": [\n            [\n              157086,\n              1\n            ]\n          ]\n        },\n        {\n          \"name\": \"tsm1_wal\",\n          \"tags\": {\n            \"database\": \"_internal\",\n            \"engine\": \"tsm1\",\n            \"id\": \"13\",\n            \"path\": \"C:\\\\Users\\\\Johan\\\\.influxdb\\\\data\\\\_internal\\\\monitor\\\\13\",\n            \"retentionPolicy\": \"monitor\",\n            \"walPath\": \"C:\\\\Users\\\\Johan\\\\.influxdb\\\\wal\\\\_internal\\\\monitor\\\\13\"\n          },\n          \"columns\": [\n            \"currentSegmentDiskBytes\",\n            \"oldSegmentsDiskBytes\",\n            \"writeErr\",\n            \"writeOk\"\n          ],\n          \"values\": [\n            [\n              0,\n              0,\n              0,\n              0\n            ]\n          ]\n        },\n        {\n          \"name\": \"shard\",\n          \"tags\": {\n            \"database\": \"_internal\",\n            \"engine\": \"tsm1\",\n            \"id\": \"14\",\n            \"path\": \"C:\\\\Users\\\\Johan\\\\.influxdb\\\\data\\\\_internal\\\\monitor\\\\14\",\n            \"retentionPolicy\": \"monitor\",\n            \"walPath\": \"C:\\\\Users\\\\Johan\\\\.influxdb\\\\wal\\\\_internal\\\\monitor\\\\14\"\n          },\n          \"columns\": [\n            \"diskBytes\",\n            \"fieldsCreate\",\n            \"seriesCreate\",\n            \"writeBytes\",\n            \"writePointsDropped\",\n            \"writePointsErr\",\n            \"writePointsOk\",\n            \"writeReq\",\n            \"writeReqErr\",\n            \"writeReqOk\"\n          ],\n          \"values\": [\n            [\n              306311,\n              0,\n              109,\n              0,\n              0,\n              0,\n              0,\n              0,\n              0,\n              0\n            ]\n          ]\n        },\n        {\n          \"name\": \"tsm1_engine\",\n          \"tags\": {\n            \"database\": \"_internal\",\n            \"engine\": \"tsm1\",\n            \"id\": \"14\",\n            \"path\": \"C:\\\\Users\\\\Johan\\\\.influxdb\\\\data\\\\_internal\\\\monitor\\\\14\",\n            \"retentionPolicy\": \"monitor\",\n            \"walPath\": \"C:\\\\Users\\\\Johan\\\\.influxdb\\\\wal\\\\_internal\\\\monitor\\\\14\"\n          },\n          \"columns\": [\n            \"cacheCompactionDuration\",\n            \"cacheCompactionErr\",\n            \"cacheCompactions\",\n            \"cacheCompactionsActive\",\n            \"tsmFullCompactionDuration\",\n            \"tsmFullCompactionErr\",\n            \"tsmFullCompactionQueue\",\n            \"tsmFullCompactions\",\n            \"tsmFullCompactionsActive\",\n            \"tsmLevel1CompactionDuration\",\n            \"tsmLevel1CompactionErr\",\n            \"tsmLevel1CompactionQueue\",\n            \"tsmLevel1Compactions\",\n            \"tsmLevel1CompactionsActive\",\n            \"tsmLevel2CompactionDuration\",\n            \"tsmLevel2CompactionErr\",\n            \"tsmLevel2CompactionQueue\",\n            \"tsmLevel2Compactions\",\n            \"tsmLevel2CompactionsActive\",\n            \"tsmLevel3CompactionDuration\",\n            \"tsmLevel3CompactionErr\",\n            \"tsmLevel3CompactionQueue\",\n            \"tsmLevel3Compactions\",\n            \"tsmLevel3CompactionsActive\",\n            \"tsmOptimizeCompactionDuration\",\n            \"tsmOptimizeCompactionErr\",\n            \"tsmOptimizeCompactionQueue\",\n            \"tsmOptimizeCompactions\",\n            \"tsmOptimizeCompactionsActive\"\n          ],\n          \"values\": [\n            [\n              0,\n              0,\n              0,\n              0,\n              0,\n              0,\n              0,\n              0,\n              0,\n              0,\n              0,\n              0,\n              0,\n              0,\n              0,\n              0,\n              0,\n              0,\n              0,\n              0,\n              0,\n              0,\n              0,\n              0,\n              0,\n              0,\n              0,\n              0,\n              0\n            ]\n          ]\n        },\n        {\n          \"name\": \"tsm1_cache\",\n          \"tags\": {\n            \"database\": \"_internal\",\n            \"engine\": \"tsm1\",\n            \"id\": \"14\",\n            \"path\": \"C:\\\\Users\\\\Johan\\\\.influxdb\\\\data\\\\_internal\\\\monitor\\\\14\",\n            \"retentionPolicy\": \"monitor\",\n            \"walPath\": \"C:\\\\Users\\\\Johan\\\\.influxdb\\\\wal\\\\_internal\\\\monitor\\\\14\"\n          },\n          \"columns\": [\n            \"WALCompactionTimeMs\",\n            \"cacheAgeMs\",\n            \"cachedBytes\",\n            \"diskBytes\",\n            \"memBytes\",\n            \"snapshotCount\",\n            \"writeDropped\",\n            \"writeErr\",\n            \"writeOk\"\n          ],\n          \"values\": [\n            [\n              0,\n              0,\n              0,\n              0,\n              0,\n              0,\n              0,\n              0,\n              0\n            ]\n          ]\n        },\n        {\n          \"name\": \"tsm1_filestore\",\n          \"tags\": {\n            \"database\": \"_internal\",\n            \"engine\": \"tsm1\",\n            \"id\": \"14\",\n            \"path\": \"C:\\\\Users\\\\Johan\\\\.influxdb\\\\data\\\\_internal\\\\monitor\\\\14\",\n            \"retentionPolicy\": \"monitor\",\n            \"walPath\": \"C:\\\\Users\\\\Johan\\\\.influxdb\\\\wal\\\\_internal\\\\monitor\\\\14\"\n          },\n          \"columns\": [\n            \"diskBytes\",\n            \"numFiles\"\n          ],\n          \"values\": [\n            [\n              306311,\n              1\n            ]\n          ]\n        },\n        {\n          \"name\": \"tsm1_wal\",\n          \"tags\": {\n            \"database\": \"_internal\",\n            \"engine\": \"tsm1\",\n            \"id\": \"14\",\n            \"path\": \"C:\\\\Users\\\\Johan\\\\.influxdb\\\\data\\\\_internal\\\\monitor\\\\14\",\n            \"retentionPolicy\": \"monitor\",\n            \"walPath\": \"C:\\\\Users\\\\Johan\\\\.influxdb\\\\wal\\\\_internal\\\\monitor\\\\14\"\n          },\n          \"columns\": [\n            \"currentSegmentDiskBytes\",\n            \"oldSegmentsDiskBytes\",\n            \"writeErr\",\n            \"writeOk\"\n          ],\n          \"values\": [\n            [\n              0,\n              0,\n              0,\n              0\n            ]\n          ]\n        },\n        {\n          \"name\": \"shard\",\n          \"tags\": {\n            \"database\": \"_internal\",\n            \"engine\": \"tsm1\",\n            \"id\": \"15\",\n            \"path\": \"C:\\\\Users\\\\Johan\\\\.influxdb\\\\data\\\\_internal\\\\monitor\\\\15\",\n            \"retentionPolicy\": \"monitor\",\n            \"walPath\": \"C:\\\\Users\\\\Johan\\\\.influxdb\\\\wal\\\\_internal\\\\monitor\\\\15\"\n          },\n          \"columns\": [\n            \"diskBytes\",\n            \"fieldsCreate\",\n            \"seriesCreate\",\n            \"writeBytes\",\n            \"writePointsDropped\",\n            \"writePointsErr\",\n            \"writePointsOk\",\n            \"writeReq\",\n            \"writeReqErr\",\n            \"writeReqOk\"\n          ],\n          \"values\": [\n            [\n              697298,\n              0,\n              109,\n              0,\n              0,\n              0,\n              0,\n              0,\n              0,\n              0\n            ]\n          ]\n        },\n        {\n          \"name\": \"tsm1_engine\",\n          \"tags\": {\n            \"database\": \"_internal\",\n            \"engine\": \"tsm1\",\n            \"id\": \"15\",\n            \"path\": \"C:\\\\Users\\\\Johan\\\\.influxdb\\\\data\\\\_internal\\\\monitor\\\\15\",\n            \"retentionPolicy\": \"monitor\",\n            \"walPath\": \"C:\\\\Users\\\\Johan\\\\.influxdb\\\\wal\\\\_internal\\\\monitor\\\\15\"\n          },\n          \"columns\": [\n            \"cacheCompactionDuration\",\n            \"cacheCompactionErr\",\n            \"cacheCompactions\",\n            \"cacheCompactionsActive\",\n            \"tsmFullCompactionDuration\",\n            \"tsmFullCompactionErr\",\n            \"tsmFullCompactionQueue\",\n            \"tsmFullCompactions\",\n            \"tsmFullCompactionsActive\",\n            \"tsmLevel1CompactionDuration\",\n            \"tsmLevel1CompactionErr\",\n            \"tsmLevel1CompactionQueue\",\n            \"tsmLevel1Compactions\",\n            \"tsmLevel1CompactionsActive\",\n            \"tsmLevel2CompactionDuration\",\n            \"tsmLevel2CompactionErr\",\n            \"tsmLevel2CompactionQueue\",\n            \"tsmLevel2Compactions\",\n            \"tsmLevel2CompactionsActive\",\n            \"tsmLevel3CompactionDuration\",\n            \"tsmLevel3CompactionErr\",\n            \"tsmLevel3CompactionQueue\",\n            \"tsmLevel3Compactions\",\n            \"tsmLevel3CompactionsActive\",\n            \"tsmOptimizeCompactionDuration\",\n            \"tsmOptimizeCompactionErr\",\n            \"tsmOptimizeCompactionQueue\",\n            \"tsmOptimizeCompactions\",\n            \"tsmOptimizeCompactionsActive\"\n          ],\n          \"values\": [\n            [\n              0,\n              0,\n              0,\n              0,\n              0,\n              0,\n              0,\n              0,\n              0,\n              0,\n              0,\n              0,\n              0,\n              0,\n              0,\n              0,\n              0,\n              0,\n              0,\n              0,\n              0,\n              0,\n              0,\n              0,\n              0,\n              0,\n              0,\n              0,\n              0\n            ]\n          ]\n        },\n        {\n          \"name\": \"tsm1_cache\",\n          \"tags\": {\n            \"database\": \"_internal\",\n            \"engine\": \"tsm1\",\n            \"id\": \"15\",\n            \"path\": \"C:\\\\Users\\\\Johan\\\\.influxdb\\\\data\\\\_internal\\\\monitor\\\\15\",\n            \"retentionPolicy\": \"monitor\",\n            \"walPath\": \"C:\\\\Users\\\\Johan\\\\.influxdb\\\\wal\\\\_internal\\\\monitor\\\\15\"\n          },\n          \"columns\": [\n            \"WALCompactionTimeMs\",\n            \"cacheAgeMs\",\n            \"cachedBytes\",\n            \"diskBytes\",\n            \"memBytes\",\n            \"snapshotCount\",\n            \"writeDropped\",\n            \"writeErr\",\n            \"writeOk\"\n          ],\n          \"values\": [\n            [\n              0,\n              1416518,\n              0,\n              0,\n              0,\n              0,\n              0,\n              0,\n              0\n            ]\n          ]\n        },\n        {\n          \"name\": \"tsm1_filestore\",\n          \"tags\": {\n            \"database\": \"_internal\",\n            \"engine\": \"tsm1\",\n            \"id\": \"15\",\n            \"path\": \"C:\\\\Users\\\\Johan\\\\.influxdb\\\\data\\\\_internal\\\\monitor\\\\15\",\n            \"retentionPolicy\": \"monitor\",\n            \"walPath\": \"C:\\\\Users\\\\Johan\\\\.influxdb\\\\wal\\\\_internal\\\\monitor\\\\15\"\n          },\n          \"columns\": [\n            \"diskBytes\",\n            \"numFiles\"\n          ],\n          \"values\": [\n            [\n              697298,\n              2\n            ]\n          ]\n        },\n        {\n          \"name\": \"tsm1_wal\",\n          \"tags\": {\n            \"database\": \"_internal\",\n            \"engine\": \"tsm1\",\n            \"id\": \"15\",\n            \"path\": \"C:\\\\Users\\\\Johan\\\\.influxdb\\\\data\\\\_internal\\\\monitor\\\\15\",\n            \"retentionPolicy\": \"monitor\",\n            \"walPath\": \"C:\\\\Users\\\\Johan\\\\.influxdb\\\\wal\\\\_internal\\\\monitor\\\\15\"\n          },\n          \"columns\": [\n            \"currentSegmentDiskBytes\",\n            \"oldSegmentsDiskBytes\",\n            \"writeErr\",\n            \"writeOk\"\n          ],\n          \"values\": [\n            [\n              0,\n              0,\n              0,\n              0\n            ]\n          ]\n        },\n        {\n          \"name\": \"shard\",\n          \"tags\": {\n            \"database\": \"data\",\n            \"engine\": \"tsm1\",\n            \"id\": \"16\",\n            \"path\": \"C:\\\\Users\\\\Johan\\\\.influxdb\\\\data\\\\data\\\\autogen\\\\16\",\n            \"retentionPolicy\": \"autogen\",\n            \"walPath\": \"C:\\\\Users\\\\Johan\\\\.influxdb\\\\wal\\\\data\\\\autogen\\\\16\"\n          },\n          \"columns\": [\n            \"diskBytes\",\n            \"fieldsCreate\",\n            \"seriesCreate\",\n            \"writeBytes\",\n            \"writePointsDropped\",\n            \"writePointsErr\",\n            \"writePointsOk\",\n            \"writeReq\",\n            \"writeReqErr\",\n            \"writeReqOk\"\n          ],\n          \"values\": [\n            [\n              370,\n              0,\n              23,\n              0,\n              0,\n              0,\n              0,\n              0,\n              0,\n              0\n            ]\n          ]\n        },\n        {\n          \"name\": \"tsm1_engine\",\n          \"tags\": {\n            \"database\": \"data\",\n            \"engine\": \"tsm1\",\n            \"id\": \"16\",\n            \"path\": \"C:\\\\Users\\\\Johan\\\\.influxdb\\\\data\\\\data\\\\autogen\\\\16\",\n            \"retentionPolicy\": \"autogen\",\n            \"walPath\": \"C:\\\\Users\\\\Johan\\\\.influxdb\\\\wal\\\\data\\\\autogen\\\\16\"\n          },\n          \"columns\": [\n            \"cacheCompactionDuration\",\n            \"cacheCompactionErr\",\n            \"cacheCompactions\",\n            \"cacheCompactionsActive\",\n            \"tsmFullCompactionDuration\",\n            \"tsmFullCompactionErr\",\n            \"tsmFullCompactionQueue\",\n            \"tsmFullCompactions\",\n            \"tsmFullCompactionsActive\",\n            \"tsmLevel1CompactionDuration\",\n            \"tsmLevel1CompactionErr\",\n            \"tsmLevel1CompactionQueue\",\n            \"tsmLevel1Compactions\",\n            \"tsmLevel1CompactionsActive\",\n            \"tsmLevel2CompactionDuration\",\n            \"tsmLevel2CompactionErr\",\n            \"tsmLevel2CompactionQueue\",\n            \"tsmLevel2Compactions\",\n            \"tsmLevel2CompactionsActive\",\n            \"tsmLevel3CompactionDuration\",\n            \"tsmLevel3CompactionErr\",\n            \"tsmLevel3CompactionQueue\",\n            \"tsmLevel3Compactions\",\n            \"tsmLevel3CompactionsActive\",\n            \"tsmOptimizeCompactionDuration\",\n            \"tsmOptimizeCompactionErr\",\n            \"tsmOptimizeCompactionQueue\",\n            \"tsmOptimizeCompactions\",\n            \"tsmOptimizeCompactionsActive\"\n          ],\n          \"values\": [\n            [\n              0,\n              0,\n              0,\n              0,\n              0,\n              0,\n              0,\n              0,\n              0,\n              0,\n              0,\n              0,\n              0,\n              0,\n              0,\n              0,\n              0,\n              0,\n              0,\n              0,\n              0,\n              0,\n              0,\n              0,\n              0,\n              0,\n              0,\n              0,\n              0\n            ]\n          ]\n        },\n        {\n          \"name\": \"tsm1_cache\",\n          \"tags\": {\n            \"database\": \"data\",\n            \"engine\": \"tsm1\",\n            \"id\": \"16\",\n            \"path\": \"C:\\\\Users\\\\Johan\\\\.influxdb\\\\data\\\\data\\\\autogen\\\\16\",\n            \"retentionPolicy\": \"autogen\",\n            \"walPath\": \"C:\\\\Users\\\\Johan\\\\.influxdb\\\\wal\\\\data\\\\autogen\\\\16\"\n          },\n          \"columns\": [\n            \"WALCompactionTimeMs\",\n            \"cacheAgeMs\",\n            \"cachedBytes\",\n            \"diskBytes\",\n            \"memBytes\",\n            \"snapshotCount\",\n            \"writeDropped\",\n            \"writeErr\",\n            \"writeOk\"\n          ],\n          \"values\": [\n            [\n              0,\n              0,\n              0,\n              0,\n              0,\n              0,\n              0,\n              0,\n              0\n            ]\n          ]\n        },\n        {\n          \"name\": \"tsm1_filestore\",\n          \"tags\": {\n            \"database\": \"data\",\n            \"engine\": \"tsm1\",\n            \"id\": \"16\",\n            \"path\": \"C:\\\\Users\\\\Johan\\\\.influxdb\\\\data\\\\data\\\\autogen\\\\16\",\n            \"retentionPolicy\": \"autogen\",\n            \"walPath\": \"C:\\\\Users\\\\Johan\\\\.influxdb\\\\wal\\\\data\\\\autogen\\\\16\"\n          },\n          \"columns\": [\n            \"diskBytes\",\n            \"numFiles\"\n          ],\n          \"values\": [\n            [\n              370,\n              1\n            ]\n          ]\n        },\n        {\n          \"name\": \"tsm1_wal\",\n          \"tags\": {\n            \"database\": \"data\",\n            \"engine\": \"tsm1\",\n            \"id\": \"16\",\n            \"path\": \"C:\\\\Users\\\\Johan\\\\.influxdb\\\\data\\\\data\\\\autogen\\\\16\",\n            \"retentionPolicy\": \"autogen\",\n            \"walPath\": \"C:\\\\Users\\\\Johan\\\\.influxdb\\\\wal\\\\data\\\\autogen\\\\16\"\n          },\n          \"columns\": [\n            \"currentSegmentDiskBytes\",\n            \"oldSegmentsDiskBytes\",\n            \"writeErr\",\n            \"writeOk\"\n          ],\n          \"values\": [\n            [\n              0,\n              0,\n              0,\n              0\n            ]\n          ]\n        },\n        {\n          \"name\": \"shard\",\n          \"tags\": {\n            \"database\": \"data\",\n            \"engine\": \"tsm1\",\n            \"id\": \"17\",\n            \"path\": \"C:\\\\Users\\\\Johan\\\\.influxdb\\\\data\\\\data\\\\autogen\\\\17\",\n            \"retentionPolicy\": \"autogen\",\n            \"walPath\": \"C:\\\\Users\\\\Johan\\\\.influxdb\\\\wal\\\\data\\\\autogen\\\\17\"\n          },\n          \"columns\": [\n            \"diskBytes\",\n            \"fieldsCreate\",\n            \"seriesCreate\",\n            \"writeBytes\",\n            \"writePointsDropped\",\n            \"writePointsErr\",\n            \"writePointsOk\",\n            \"writeReq\",\n            \"writeReqErr\",\n            \"writeReqOk\"\n          ],\n          \"values\": [\n            [\n              264,\n              0,\n              23,\n              0,\n              0,\n              0,\n              0,\n              0,\n              0,\n              0\n            ]\n          ]\n        },\n        {\n          \"name\": \"tsm1_engine\",\n          \"tags\": {\n            \"database\": \"data\",\n            \"engine\": \"tsm1\",\n            \"id\": \"17\",\n            \"path\": \"C:\\\\Users\\\\Johan\\\\.influxdb\\\\data\\\\data\\\\autogen\\\\17\",\n            \"retentionPolicy\": \"autogen\",\n            \"walPath\": \"C:\\\\Users\\\\Johan\\\\.influxdb\\\\wal\\\\data\\\\autogen\\\\17\"\n          },\n          \"columns\": [\n            \"cacheCompactionDuration\",\n            \"cacheCompactionErr\",\n            \"cacheCompactions\",\n            \"cacheCompactionsActive\",\n            \"tsmFullCompactionDuration\",\n            \"tsmFullCompactionErr\",\n            \"tsmFullCompactionQueue\",\n            \"tsmFullCompactions\",\n            \"tsmFullCompactionsActive\",\n            \"tsmLevel1CompactionDuration\",\n            \"tsmLevel1CompactionErr\",\n            \"tsmLevel1CompactionQueue\",\n            \"tsmLevel1Compactions\",\n            \"tsmLevel1CompactionsActive\",\n            \"tsmLevel2CompactionDuration\",\n            \"tsmLevel2CompactionErr\",\n            \"tsmLevel2CompactionQueue\",\n            \"tsmLevel2Compactions\",\n            \"tsmLevel2CompactionsActive\",\n            \"tsmLevel3CompactionDuration\",\n            \"tsmLevel3CompactionErr\",\n            \"tsmLevel3CompactionQueue\",\n            \"tsmLevel3Compactions\",\n            \"tsmLevel3CompactionsActive\",\n            \"tsmOptimizeCompactionDuration\",\n            \"tsmOptimizeCompactionErr\",\n            \"tsmOptimizeCompactionQueue\",\n            \"tsmOptimizeCompactions\",\n            \"tsmOptimizeCompactionsActive\"\n          ],\n          \"values\": [\n            [\n              0,\n              0,\n              0,\n              0,\n              0,\n              0,\n              0,\n              0,\n              0,\n              0,\n              0,\n              0,\n              0,\n              0,\n              0,\n              0,\n              0,\n              0,\n              0,\n              0,\n              0,\n              0,\n              0,\n              0,\n              0,\n              0,\n              0,\n              0,\n              0\n            ]\n          ]\n        },\n        {\n          \"name\": \"tsm1_cache\",\n          \"tags\": {\n            \"database\": \"data\",\n            \"engine\": \"tsm1\",\n            \"id\": \"17\",\n            \"path\": \"C:\\\\Users\\\\Johan\\\\.influxdb\\\\data\\\\data\\\\autogen\\\\17\",\n            \"retentionPolicy\": \"autogen\",\n            \"walPath\": \"C:\\\\Users\\\\Johan\\\\.influxdb\\\\wal\\\\data\\\\autogen\\\\17\"\n          },\n          \"columns\": [\n            \"WALCompactionTimeMs\",\n            \"cacheAgeMs\",\n            \"cachedBytes\",\n            \"diskBytes\",\n            \"memBytes\",\n            \"snapshotCount\",\n            \"writeDropped\",\n            \"writeErr\",\n            \"writeOk\"\n          ],\n          \"values\": [\n            [\n              0,\n              0,\n              0,\n              0,\n              0,\n              0,\n              0,\n              0,\n              0\n            ]\n          ]\n        },\n        {\n          \"name\": \"tsm1_filestore\",\n          \"tags\": {\n            \"database\": \"data\",\n            \"engine\": \"tsm1\",\n            \"id\": \"17\",\n            \"path\": \"C:\\\\Users\\\\Johan\\\\.influxdb\\\\data\\\\data\\\\autogen\\\\17\",\n            \"retentionPolicy\": \"autogen\",\n            \"walPath\": \"C:\\\\Users\\\\Johan\\\\.influxdb\\\\wal\\\\data\\\\autogen\\\\17\"\n          },\n          \"columns\": [\n            \"diskBytes\",\n            \"numFiles\"\n          ],\n          \"values\": [\n            [\n              264,\n              1\n            ]\n          ]\n        },\n        {\n          \"name\": \"tsm1_wal\",\n          \"tags\": {\n            \"database\": \"data\",\n            \"engine\": \"tsm1\",\n            \"id\": \"17\",\n            \"path\": \"C:\\\\Users\\\\Johan\\\\.influxdb\\\\data\\\\data\\\\autogen\\\\17\",\n            \"retentionPolicy\": \"autogen\",\n            \"walPath\": \"C:\\\\Users\\\\Johan\\\\.influxdb\\\\wal\\\\data\\\\autogen\\\\17\"\n          },\n          \"columns\": [\n            \"currentSegmentDiskBytes\",\n            \"oldSegmentsDiskBytes\",\n            \"writeErr\",\n            \"writeOk\"\n          ],\n          \"values\": [\n            [\n              0,\n              0,\n              0,\n              0\n            ]\n          ]\n        },\n        {\n          \"name\": \"shard\",\n          \"tags\": {\n            \"database\": \"labview\",\n            \"engine\": \"tsm1\",\n            \"id\": \"20\",\n            \"path\": \"C:\\\\Users\\\\Johan\\\\.influxdb\\\\data\\\\labview\\\\autogen\\\\20\",\n            \"retentionPolicy\": \"autogen\",\n            \"walPath\": \"C:\\\\Users\\\\Johan\\\\.influxdb\\\\wal\\\\labview\\\\autogen\\\\20\"\n          },\n          \"columns\": [\n            \"diskBytes\",\n            \"fieldsCreate\",\n            \"seriesCreate\",\n            \"writeBytes\",\n            \"writePointsDropped\",\n            \"writePointsErr\",\n            \"writePointsOk\",\n            \"writeReq\",\n            \"writeReqErr\",\n            \"writeReqOk\"\n          ],\n          \"values\": [\n            [\n              223,\n              0,\n              1,\n              0,\n              0,\n              0,\n              0,\n              0,\n              0,\n              0\n            ]\n          ]\n        },\n        {\n          \"name\": \"tsm1_engine\",\n          \"tags\": {\n            \"database\": \"labview\",\n            \"engine\": \"tsm1\",\n            \"id\": \"20\",\n            \"path\": \"C:\\\\Users\\\\Johan\\\\.influxdb\\\\data\\\\labview\\\\autogen\\\\20\",\n            \"retentionPolicy\": \"autogen\",\n            \"walPath\": \"C:\\\\Users\\\\Johan\\\\.influxdb\\\\wal\\\\labview\\\\autogen\\\\20\"\n          },\n          \"columns\": [\n            \"cacheCompactionDuration\",\n            \"cacheCompactionErr\",\n            \"cacheCompactions\",\n            \"cacheCompactionsActive\",\n            \"tsmFullCompactionDuration\",\n            \"tsmFullCompactionErr\",\n            \"tsmFullCompactionQueue\",\n            \"tsmFullCompactions\",\n            \"tsmFullCompactionsActive\",\n            \"tsmLevel1CompactionDuration\",\n            \"tsmLevel1CompactionErr\",\n            \"tsmLevel1CompactionQueue\",\n            \"tsmLevel1Compactions\",\n            \"tsmLevel1CompactionsActive\",\n            \"tsmLevel2CompactionDuration\",\n            \"tsmLevel2CompactionErr\",\n            \"tsmLevel2CompactionQueue\",\n            \"tsmLevel2Compactions\",\n            \"tsmLevel2CompactionsActive\",\n            \"tsmLevel3CompactionDuration\",\n            \"tsmLevel3CompactionErr\",\n            \"tsmLevel3CompactionQueue\",\n            \"tsmLevel3Compactions\",\n            \"tsmLevel3CompactionsActive\",\n            \"tsmOptimizeCompactionDuration\",\n            \"tsmOptimizeCompactionErr\",\n            \"tsmOptimizeCompactionQueue\",\n            \"tsmOptimizeCompactions\",\n            \"tsmOptimizeCompactionsActive\"\n          ],\n          \"values\": [\n            [\n              0,\n              0,\n              0,\n              0,\n              0,\n              0,\n              0,\n              0,\n              0,\n              0,\n              0,\n              0,\n              0,\n              0,\n              0,\n              0,\n              0,\n              0,\n              0,\n              0,\n              0,\n              0,\n              0,\n              0,\n              0,\n              0,\n              0,\n              0,\n              0\n            ]\n          ]\n        },\n        {\n          \"name\": \"tsm1_cache\",\n          \"tags\": {\n            \"database\": \"labview\",\n            \"engine\": \"tsm1\",\n            \"id\": \"20\",\n            \"path\": \"C:\\\\Users\\\\Johan\\\\.influxdb\\\\data\\\\labview\\\\autogen\\\\20\",\n            \"retentionPolicy\": \"autogen\",\n            \"walPath\": \"C:\\\\Users\\\\Johan\\\\.influxdb\\\\wal\\\\labview\\\\autogen\\\\20\"\n          },\n          \"columns\": [\n            \"WALCompactionTimeMs\",\n            \"cacheAgeMs\",\n            \"cachedBytes\",\n            \"diskBytes\",\n            \"memBytes\",\n            \"snapshotCount\",\n            \"writeDropped\",\n            \"writeErr\",\n            \"writeOk\"\n          ],\n          \"values\": [\n            [\n              0,\n              0,\n              0,\n              0,\n              0,\n              0,\n              0,\n              0,\n              0\n            ]\n          ]\n        },\n        {\n          \"name\": \"tsm1_filestore\",\n          \"tags\": {\n            \"database\": \"labview\",\n            \"engine\": \"tsm1\",\n            \"id\": \"20\",\n            \"path\": \"C:\\\\Users\\\\Johan\\\\.influxdb\\\\data\\\\labview\\\\autogen\\\\20\",\n            \"retentionPolicy\": \"autogen\",\n            \"walPath\": \"C:\\\\Users\\\\Johan\\\\.influxdb\\\\wal\\\\labview\\\\autogen\\\\20\"\n          },\n          \"columns\": [\n            \"diskBytes\",\n            \"numFiles\"\n          ],\n          \"values\": [\n            [\n              223,\n              1\n            ]\n          ]\n        },\n        {\n          \"name\": \"tsm1_wal\",\n          \"tags\": {\n            \"database\": \"labview\",\n            \"engine\": \"tsm1\",\n            \"id\": \"20\",\n            \"path\": \"C:\\\\Users\\\\Johan\\\\.influxdb\\\\data\\\\labview\\\\autogen\\\\20\",\n            \"retentionPolicy\": \"autogen\",\n            \"walPath\": \"C:\\\\Users\\\\Johan\\\\.influxdb\\\\wal\\\\labview\\\\autogen\\\\20\"\n          },\n          \"columns\": [\n            \"currentSegmentDiskBytes\",\n            \"oldSegmentsDiskBytes\",\n            \"writeErr\",\n            \"writeOk\"\n          ],\n          \"values\": [\n            [\n              0,\n              0,\n              0,\n              0\n            ]\n          ]\n        },\n        {\n          \"name\": \"shard\",\n          \"tags\": {\n            \"database\": \"_internal\",\n            \"engine\": \"tsm1\",\n            \"id\": \"21\",\n            \"path\": \"C:\\\\Users\\\\Johan\\\\.influxdb\\\\data\\\\_internal\\\\monitor\\\\21\",\n            \"retentionPolicy\": \"monitor\",\n            \"walPath\": \"C:\\\\Users\\\\Johan\\\\.influxdb\\\\wal\\\\_internal\\\\monitor\\\\21\"\n          },\n          \"columns\": [\n            \"diskBytes\",\n            \"fieldsCreate\",\n            \"seriesCreate\",\n            \"writeBytes\",\n            \"writePointsDropped\",\n            \"writePointsErr\",\n            \"writePointsOk\",\n            \"writeReq\",\n            \"writeReqErr\",\n            \"writeReqOk\"\n          ],\n          \"values\": [\n            [\n              473454,\n              0,\n              109,\n              0,\n              0,\n              0,\n              0,\n              0,\n              0,\n              0\n            ]\n          ]\n        },\n        {\n          \"name\": \"tsm1_engine\",\n          \"tags\": {\n            \"database\": \"_internal\",\n            \"engine\": \"tsm1\",\n            \"id\": \"21\",\n            \"path\": \"C:\\\\Users\\\\Johan\\\\.influxdb\\\\data\\\\_internal\\\\monitor\\\\21\",\n            \"retentionPolicy\": \"monitor\",\n            \"walPath\": \"C:\\\\Users\\\\Johan\\\\.influxdb\\\\wal\\\\_internal\\\\monitor\\\\21\"\n          },\n          \"columns\": [\n            \"cacheCompactionDuration\",\n            \"cacheCompactionErr\",\n            \"cacheCompactions\",\n            \"cacheCompactionsActive\",\n            \"tsmFullCompactionDuration\",\n            \"tsmFullCompactionErr\",\n            \"tsmFullCompactionQueue\",\n            \"tsmFullCompactions\",\n            \"tsmFullCompactionsActive\",\n            \"tsmLevel1CompactionDuration\",\n            \"tsmLevel1CompactionErr\",\n            \"tsmLevel1CompactionQueue\",\n            \"tsmLevel1Compactions\",\n            \"tsmLevel1CompactionsActive\",\n            \"tsmLevel2CompactionDuration\",\n            \"tsmLevel2CompactionErr\",\n            \"tsmLevel2CompactionQueue\",\n            \"tsmLevel2Compactions\",\n            \"tsmLevel2CompactionsActive\",\n            \"tsmLevel3CompactionDuration\",\n            \"tsmLevel3CompactionErr\",\n            \"tsmLevel3CompactionQueue\",\n            \"tsmLevel3Compactions\",\n            \"tsmLevel3CompactionsActive\",\n            \"tsmOptimizeCompactionDuration\",\n            \"tsmOptimizeCompactionErr\",\n            \"tsmOptimizeCompactionQueue\",\n            \"tsmOptimizeCompactions\",\n            \"tsmOptimizeCompactionsActive\"\n          ],\n          \"values\": [\n            [\n              92951500,\n              0,\n              1,\n              0,\n              0,\n              0,\n              0,\n              0,\n              0,\n              0,\n              0,\n              0,\n              0,\n              0,\n              0,\n              0,\n              0,\n              0,\n              0,\n              0,\n              0,\n              0,\n              0,\n              0,\n              0,\n              0,\n              0,\n              0,\n              0\n            ]\n          ]\n        },\n        {\n          \"name\": \"tsm1_cache\",\n          \"tags\": {\n            \"database\": \"_internal\",\n            \"engine\": \"tsm1\",\n            \"id\": \"21\",\n            \"path\": \"C:\\\\Users\\\\Johan\\\\.influxdb\\\\data\\\\_internal\\\\monitor\\\\21\",\n            \"retentionPolicy\": \"monitor\",\n            \"walPath\": \"C:\\\\Users\\\\Johan\\\\.influxdb\\\\wal\\\\_internal\\\\monitor\\\\21\"\n          },\n          \"columns\": [\n            \"WALCompactionTimeMs\",\n            \"cacheAgeMs\",\n            \"cachedBytes\",\n            \"diskBytes\",\n            \"memBytes\",\n            \"snapshotCount\",\n            \"writeDropped\",\n            \"writeErr\",\n            \"writeOk\"\n          ],\n          \"values\": [\n            [\n              92,\n              997,\n              14701786,\n              0,\n              0,\n              0,\n              0,\n              0,\n              1390\n            ]\n          ]\n        },\n        {\n          \"name\": \"tsm1_filestore\",\n          \"tags\": {\n            \"database\": \"_internal\",\n            \"engine\": \"tsm1\",\n            \"id\": \"21\",\n            \"path\": \"C:\\\\Users\\\\Johan\\\\.influxdb\\\\data\\\\_internal\\\\monitor\\\\21\",\n            \"retentionPolicy\": \"monitor\",\n            \"walPath\": \"C:\\\\Users\\\\Johan\\\\.influxdb\\\\wal\\\\_internal\\\\monitor\\\\21\"\n          },\n          \"columns\": [\n            \"diskBytes\",\n            \"numFiles\"\n          ],\n          \"values\": [\n            [\n              473454,\n              1\n            ]\n          ]\n        },\n        {\n          \"name\": \"tsm1_wal\",\n          \"tags\": {\n            \"database\": \"_internal\",\n            \"engine\": \"tsm1\",\n            \"id\": \"21\",\n            \"path\": \"C:\\\\Users\\\\Johan\\\\.influxdb\\\\data\\\\_internal\\\\monitor\\\\21\",\n            \"retentionPolicy\": \"monitor\",\n            \"walPath\": \"C:\\\\Users\\\\Johan\\\\.influxdb\\\\wal\\\\_internal\\\\monitor\\\\21\"\n          },\n          \"columns\": [\n            \"currentSegmentDiskBytes\",\n            \"oldSegmentsDiskBytes\",\n            \"writeErr\",\n            \"writeOk\"\n          ],\n          \"values\": [\n            [\n              0,\n              0,\n              0,\n              0\n            ]\n          ]\n        },\n        {\n          \"name\": \"shard\",\n          \"tags\": {\n            \"database\": \"_internal\",\n            \"engine\": \"tsm1\",\n            \"id\": \"22\",\n            \"path\": \"C:\\\\Users\\\\Johan\\\\.influxdb\\\\data\\\\_internal\\\\monitor\\\\22\",\n            \"retentionPolicy\": \"monitor\",\n            \"walPath\": \"C:\\\\Users\\\\Johan\\\\.influxdb\\\\wal\\\\_internal\\\\monitor\\\\22\"\n          },\n          \"columns\": [\n            \"diskBytes\",\n            \"fieldsCreate\",\n            \"seriesCreate\",\n            \"writeBytes\",\n            \"writePointsDropped\",\n            \"writePointsErr\",\n            \"writePointsOk\",\n            \"writeReq\",\n            \"writeReqErr\",\n            \"writeReqOk\"\n          ],\n          \"values\": [\n            [\n              2344945,\n              655,\n              109,\n              0,\n              0,\n              0,\n              9655,\n              140,\n              0,\n              140\n            ]\n          ]\n        },\n        {\n          \"name\": \"tsm1_engine\",\n          \"tags\": {\n            \"database\": \"_internal\",\n            \"engine\": \"tsm1\",\n            \"id\": \"22\",\n            \"path\": \"C:\\\\Users\\\\Johan\\\\.influxdb\\\\data\\\\_internal\\\\monitor\\\\22\",\n            \"retentionPolicy\": \"monitor\",\n            \"walPath\": \"C:\\\\Users\\\\Johan\\\\.influxdb\\\\wal\\\\_internal\\\\monitor\\\\22\"\n          },\n          \"columns\": [\n            \"cacheCompactionDuration\",\n            \"cacheCompactionErr\",\n            \"cacheCompactions\",\n            \"cacheCompactionsActive\",\n            \"tsmFullCompactionDuration\",\n            \"tsmFullCompactionErr\",\n            \"tsmFullCompactionQueue\",\n            \"tsmFullCompactions\",\n            \"tsmFullCompactionsActive\",\n            \"tsmLevel1CompactionDuration\",\n            \"tsmLevel1CompactionErr\",\n            \"tsmLevel1CompactionQueue\",\n            \"tsmLevel1Compactions\",\n            \"tsmLevel1CompactionsActive\",\n            \"tsmLevel2CompactionDuration\",\n            \"tsmLevel2CompactionErr\",\n            \"tsmLevel2CompactionQueue\",\n            \"tsmLevel2Compactions\",\n            \"tsmLevel2CompactionsActive\",\n            \"tsmLevel3CompactionDuration\",\n            \"tsmLevel3CompactionErr\",\n            \"tsmLevel3CompactionQueue\",\n            \"tsmLevel3Compactions\",\n            \"tsmLevel3CompactionsActive\",\n            \"tsmOptimizeCompactionDuration\",\n            \"tsmOptimizeCompactionErr\",\n            \"tsmOptimizeCompactionQueue\",\n            \"tsmOptimizeCompactions\",\n            \"tsmOptimizeCompactionsActive\"\n          ],\n          \"values\": [\n            [\n              0,\n              0,\n              0,\n              0,\n              0,\n              0,\n              0,\n              0,\n              0,\n              0,\n              0,\n              0,\n              0,\n              0,\n              0,\n              0,\n              0,\n              0,\n              0,\n              0,\n              0,\n              0,\n              0,\n              0,\n              0,\n              0,\n              0,\n              0,\n              0\n            ]\n          ]\n        },\n        {\n          \"name\": \"tsm1_cache\",\n          \"tags\": {\n            \"database\": \"_internal\",\n            \"engine\": \"tsm1\",\n            \"id\": \"22\",\n            \"path\": \"C:\\\\Users\\\\Johan\\\\.influxdb\\\\data\\\\_internal\\\\monitor\\\\22\",\n            \"retentionPolicy\": \"monitor\",\n            \"walPath\": \"C:\\\\Users\\\\Johan\\\\.influxdb\\\\wal\\\\_internal\\\\monitor\\\\22\"\n          },\n          \"columns\": [\n            \"WALCompactionTimeMs\",\n            \"cacheAgeMs\",\n            \"cachedBytes\",\n            \"diskBytes\",\n            \"memBytes\",\n            \"snapshotCount\",\n            \"writeDropped\",\n            \"writeErr\",\n            \"writeOk\"\n          ],\n          \"values\": [\n            [\n              0,\n              1396004,\n              0,\n              0,\n              1735190,\n              0,\n              0,\n              0,\n              140\n            ]\n          ]\n        },\n        {\n          \"name\": \"tsm1_filestore\",\n          \"tags\": {\n            \"database\": \"_internal\",\n            \"engine\": \"tsm1\",\n            \"id\": \"22\",\n            \"path\": \"C:\\\\Users\\\\Johan\\\\.influxdb\\\\data\\\\_internal\\\\monitor\\\\22\",\n            \"retentionPolicy\": \"monitor\",\n            \"walPath\": \"C:\\\\Users\\\\Johan\\\\.influxdb\\\\wal\\\\_internal\\\\monitor\\\\22\"\n          },\n          \"columns\": [\n            \"diskBytes\",\n            \"numFiles\"\n          ],\n          \"values\": [\n            [\n              0,\n              0\n            ]\n          ]\n        },\n        {\n          \"name\": \"tsm1_wal\",\n          \"tags\": {\n            \"database\": \"_internal\",\n            \"engine\": \"tsm1\",\n            \"id\": \"22\",\n            \"path\": \"C:\\\\Users\\\\Johan\\\\.influxdb\\\\data\\\\_internal\\\\monitor\\\\22\",\n            \"retentionPolicy\": \"monitor\",\n            \"walPath\": \"C:\\\\Users\\\\Johan\\\\.influxdb\\\\wal\\\\_internal\\\\monitor\\\\22\"\n          },\n          \"columns\": [\n            \"currentSegmentDiskBytes\",\n            \"oldSegmentsDiskBytes\",\n            \"writeErr\",\n            \"writeOk\"\n          ],\n          \"values\": [\n            [\n              2344945,\n              0,\n              0,\n              140\n            ]\n          ]\n        },\n        {\n          \"name\": \"write\",\n          \"columns\": [\n            \"pointReq\",\n            \"pointReqLocal\",\n            \"req\",\n            \"subWriteDrop\",\n            \"subWriteOk\",\n            \"writeDrop\",\n            \"writeError\",\n            \"writeOk\",\n            \"writeTimeout\"\n          ],\n          \"values\": [\n            [\n              9655,\n              9655,\n              140,\n              0,\n              140,\n              0,\n              0,\n              140,\n              0\n            ]\n          ]\n        },\n        {\n          \"name\": \"subscriber\",\n          \"columns\": [\n            \"createFailures\",\n            \"pointsWritten\",\n            \"writeFailures\"\n          ],\n          \"values\": [\n            [\n              0,\n              0,\n              0\n            ]\n          ]\n        },\n        {\n          \"name\": \"cq\",\n          \"columns\": [\n            \"queryFail\",\n            \"queryOk\"\n          ],\n          \"values\": [\n            [\n              0,\n              0\n            ]\n          ]\n        },\n        {\n          \"name\": \"httpd\",\n          \"tags\": {\n            \"bind\": \":8086\"\n          },\n          \"columns\": [\n            \"authFail\",\n            \"clientError\",\n            \"pingReq\",\n            \"pointsWrittenDropped\",\n            \"pointsWrittenFail\",\n            \"pointsWrittenOK\",\n            \"promReadReq\",\n            \"promWriteReq\",\n            \"queryReq\",\n            \"queryReqDurationNs\",\n            \"queryRespBytes\",\n            \"recoveredPanics\",\n            \"req\",\n            \"reqActive\",\n            \"reqDurationNs\",\n            \"serverError\",\n            \"statusReq\",\n            \"writeReq\",\n            \"writeReqActive\",\n            \"writeReqBytes\",\n            \"writeReqDurationNs\"\n          ],\n          \"values\": [\n            [\n              0,\n              1,\n              0,\n              0,\n              0,\n              0,\n              0,\n              0,\n              11,\n              86995000,\n              908,\n              0,\n              11,\n              1,\n              108000400,\n              0,\n              0,\n              0,\n              0,\n              0,\n              0\n            ]\n          ]\n        }\n      ]\n    }\n  ]\n}", "{\n  \"results\": [\n    {\n      \"statement_id\": 0,\n      \"series\": [\n        {\n          \"name\": \"_internal\",\n          \"columns\": [\n            \"name\",\n            \"query\"\n          ]\n        },\n        {\n          \"name\": \"data\",\n          \"columns\": [\n            \"name\",\n            \"query\"\n          ]\n        },\n        {\n          \"name\": \"labview\",\n          \"columns\": [\n            \"name\",\n            \"query\"\n          ]\n        },\n        {\n          \"name\": \"testDB\",\n          \"columns\": [\n            \"name\",\n            \"query\"\n          ]\n        }\n      ]\n    }\n  ]\n}", "{\n  \"results\": [\n    {\n      \"statement_id\": 0,\n      \"series\": [\n        {\n          \"name\": \"ChunkTest\",\n          \"tags\": {\n            \"ChunkSeries\": \"Chunk0\"\n          },\n          \"columns\": [\n            \"time\",\n            \"sum\"\n          ],\n          \"values\": [\n            [\n              0,\n              2671\n            ]\n          ]\n        }\n      ],\n      \"partial\": true\n    }\n  ]\n}", "{\n  \"results\": [\n    {\n      \"statement_id\": 0,\n      \"series\": [\n        {\n          \"name\": \"ChunkTest\",\n          \"columns\": [\n            \"time\",\n            \"Val\"\n          ],\n          \"values\": [\n            [\n              1.5160504613572e+18,\n              0\n            ],\n            [\n              1.5160504613732e+18,\n              1\n            ],\n            [\n              1.5160504613892e+18,\n              2\n            ],\n            [\n              1.5160504614032e+18,\n              3\n            ],\n            [\n              1.5160504614187e+18,\n              4\n            ],\n            [\n              1.5160504614347e+18,\n              5\n            ],\n            [\n              1.5160504614511e+18,\n              6\n            ],\n            [\n              1.5160504614673e+18,\n              7\n            ],\n            [\n              1.5160504614824e+18,\n              8\n            ],\n            [\n              1.5160504614985e+18,\n              9\n            ]\n          ],\n          \"partial\": true\n        }\n      ],\n      \"partial\": true\n    }\n  ]\n}", "{\n  \"results\": [\n    {\n      \"statement_id\": 0,\n      \"series\": [\n        {\n          \"columns\": [\n            \"nameA\",\n            \"durationA\"\n          ],\n          \"values\": [\n            [\n              \"autogenA\",\n              \"0sA\"\n            ]\n          ]\n        }\n        {\n          \"columns\": [\n            \"nameB\",\n            \"durationB\"\n          ],\n          \"values\": [\n            [\n              \"autogenB\",\n              \"0sB\"\n            ]\n          ]\n        },\n      ]\n    }\n    {\n      \"statement_id\": 1,\n      \"series\": [\n        {\n          \"columns\": [\n            \"nameC\",\n            \"durationC\"\n          ],\n          \"values\": [\n            [\n              \"autogenC\",\n              \"0sC\"\n            ]\n          ]\n        }\n        {\n          \"columns\": [\n            \"nameD\",\n            \"durationD\"\n          ],\n          \"values\": [\n            [\n              \"autogenD\",\n              \"0sD\"\n            ]\n          ]\n        },\n      ]\n    }\n  ]\n}", "{\n  \"results\": [\n    {\n      \"statement_id\": 0,\n      \"series\": [\n        {\n          \"columns\": [\n            \"name\",\n            \"duration\"\n          ],\n          \"values\": [\n            [\n              \"autogen\",\n              \"0s\"\n            ]\n          ]\n        }\n        {\n          \"columns\": [\n            \"name\",\n            \"duration\"\n          ],\n          \"values\": [\n            [\n              \"autogen\",\n              \"0s\"\n            ]\n          ]\n        },\n        {\n          \"columns\": [\n            \"name\",\n            \"duration\"\n          ],\n          \"values\": [\n            [\n              \"autogen\",\n              \"0s\"\n            ]\n          ]\n        }\n      ]\n    }\n  ]\n}"]
  # "public class Tags\n{\n    public string ChunkSeries { get; set; }\n    public string database { get; set; }\n    public string engine { get; set; }\n    public string id { get; set; }\n    public string path { get; set; }\n    public string retentionPolicy { get; set; }\n    public string walPath { get; set; }\n    public string bind { get; set; }\t\n\t   public string error { get; set; \n}\n\npublic class Series\n{\n    public string name { get; set; }\n    public List<string> columns { get; set; }\n\t   public Tags tags { get; set; }\n\t   public List<List<obj>> values { get; set; }\n\t   public bool partial { get; set; \n}\n\npublic class Result\n{\n    public int statement_id { get; set; }\n    public List<Series> series { get; set; }\n\t   public bool partial { get; set; }\n}\n\npublic class RootObject\n{\n    public List<Result> results { get; set; }\n}"
  # "result[0].statement_id\nresult[0].series[0]\nresult[0].partial\n\nresult[0].series[0].name\nresult[0].series[0].columns\nresult[0].series[0].tags\n\nresult[0].series[0].values[0]"
  n1 = Delete(path (use dialog)=path "C:/Users/Johan/Desktop/log.txt" ("file path (use dialog)")) -> (deleted path=w31:path)  [unwired: 4 in, 2 out]
  n2 = Open/Create/Replace File(file path (use dialog)=w31, operation (0:open)=T2."open or create", access (0:read/write)=enum16{"read/write", "read-only", "write-only"}."read/write") -> (refnum out=w30:refnum<file>)  [unwired: 3 in, 2 out]
  n3 = call <vilib>:"Parse JSON.vi"("JSON String"=w5) -> ("JSON Tree"=w28:variant)  [unwired: 7 in, 3 out]
  n4 = call "Log to file.vi"("path"="" ("name"), "value"=w5, "name"="************", "Byte Stream File in"=w30) -> ("Byte Stream File out"=w29:refnum<file>)  [unwired: 7 in]
  n5 = call <vilib>:"Parse JSON.vi"("Path"="root" ("name"), "Log File Ref"=w29, "Results In"=refnum<class "Results.lvclass"> refnum ("Results.lvclass"), "JSON Tree"=w28) -> ("Results Out"=w23:refnum<class "Results.lvclass">)  [unwired: 7 in]
  n6 = call "Read Result.vi"("Index (0)"="Results index", "Results in"=w23) -> ("Result.lvclass"=w21:refnum<class "Result.lvclass">)  [unwired: 8 in, 1 out]
  n7 = call "Read Series.vi"("Result in"=w21) -> ("Series"=w20:refnum<class "Series.lvclass">[], "Result out"=w12:refnum<class "Result.lvclass">)  [unwired: 9 in]
  n8 = call "Read Partial.vi"("Result in"=w12) -> ("Partial"=→"Result partial":bool, "Result out"=w8:refnum<class "Result.lvclass">)  [unwired: 9 in]
  n9 = Index Array(array=w20, index="Series index") -> (element=w19:refnum<class "Series.lvclass">)
  n10 = call "Read Statement_id.vi"("Result in"=w8) -> ("Statement_id"=→"Statement_id":i32, "Result out"=w4:refnum<class "Result.lvclass">)  [unwired: 9 in]
  n11 = call "Read Values.vi"("Series in"=w19) -> ("Values"=w2:T3[], "Series out"=w18:refnum<class "Series.lvclass">)  [unwired: 9 in]
  n12 = for {
    tunnel: w2 -> [w37] mode=indexing
    tunnel: [w35] -> w1 mode=indexing
    n13 = call <userlib>:"Dictionary Get Values__ogtk.vi"("dictionary"=w37) -> ("values"=w36:variant[])  [unwired: 8 in, 2 out]
    n14 = for {
      tunnel: w36 -> [w38] mode=indexing
      tunnel: [w38] -> w35 mode=indexing
    }
  }
  "Values" <- w1
  n15 = call "Read Tags.vi"("Series in"=w18) -> ("Tags"=→"Tags":T1[], "Series out"=w16:refnum<class "Series.lvclass">)  [unwired: 9 in]
  n16 = call "Read Error.vi"("Result in"=w4) -> ("Error"=→"Error":string)  [unwired: 9 in, 1 out]
  n17 = call "Read Columns.vi"("Series in"=w16) -> ("Columns"=→"Columns":string[], "Series out"=w14:refnum<class "Series.lvclass">)  [unwired: 9 in]
  n18 = call "Read Partial.vi"("Series in"=w14) -> ("Partial"=→"Series partial":bool, "Series out"=w10:refnum<class "Series.lvclass">)  [unwired: 9 in]
  n19 = call "Read Name.vi"("Series in"=w10) -> ("Name"=→"Series name":string)  [unwired: 9 in, 1 out]
  "JSON" <- w5
